vi "cRIO_4DOF_Admittance_control_v11_NewMousetrack.vi"() -> ()   [LabVIEW 2019]
uses:
  <vilib>/Platform/TimedLoop/XDataNode/timing_clust.ctl
  <vilib>/Platform/TimedLoop/XDataNode/nitl_modes.ctl
  <vilib>/Platform/TimedLoop/XDataNode/wakeup.ctl
  <vilib>/Analysis/baseanly.llb/Mean (DBL).vi
  Global 1.vi
  <vilib>/addons/control/pid/pid.llb/PID (DBL Array).vi
  <vilib>/imath/engines/lvmath2/RunTimeEngine/ArithmeticOperatorToken/NIMS_ArithmeticOperator_multmx(M,CV).vi
  <instcachedir>/0/NIMS_ArithmeticOperator_multmx(M,CV)_1D61EED49E1847F3B05DBB8EDD2FBF8F.lvgen/NIMS_ArithmeticOperator_multmx(M,CV)_1D61EED49E1847F3B05DBB8EDD2FBF8F_000.vi
  <vilib>/imathl/engines/lvmath/Functions/Error Handling/Create Error.vi
  <vilib>/imath/engines/lvmath2/RunTimeEngine/NodeEndStatement/NIMS_NodeEndStatement_Output.vi
  <instcachedir>/0/NIMS_NodeEndStatement_Output_53EC0D466D134D7ABD903AC30B43404B.lvgen/NIMS_NodeEndStatement_Output_53EC0D466D134D7ABD903AC30B43404B_002.vi
  <vilib>/imath/engines/lvmath2/RunTimeEngine/ErrorHandling/NIMS_Finalize Error.vi
  <instcachedir>/0/NIMS_NodeEndStatement_Output_53EC0D466D134D7ABD903AC30B43404B.lvgen/NIMS_NodeEndStatement_Output_53EC0D466D134D7ABD903AC30B43404B_001.vi
  <vilib>/imath/engines/lvmath2/RunTimeEngine/BuiltInFunctions/inv/NIMS_inv(GM).vi
  <instcachedir>/0/NIMS_inv(GM)_A6DF8FE880224208AACFE4CF9F659502.lvgen/NIMS_inv(GM)_A6DF8FE880224208AACFE4CF9F659502_000.vi
  <vilib>/imath/engines/lvmath2/RunTimeEngine/ErrorHandling/NIMS_Create Error From Enums.vi
  <vilib>/imath/engines/lvmath2/RunTimeEngine/IndexRead/NIMS M(R2,S).vi
  <instcachedir>/0/NIMS M(R2,S)_56813DCFDD5A484292D2195AF15D2BF5.lvgen/NIMS M(R2,S)_56813DCFDD5A484292D2195AF15D2BF5_000.vi
  <vilib>/imath/engines/lvmath2/RunTimeEngine/IndexRead/NIMS M(S,S).vi
  <instcachedir>/0/NIMS M(S,S)_AC51E74150A542F7991B9634C66F3096.lvgen/NIMS M(S,S)_AC51E74150A542F7991B9634C66F3096_000.vi
  <instcachedir>/0/NIMS_NodeEndStatement_Output_53EC0D466D134D7ABD903AC30B43404B.lvgen/NIMS_NodeEndStatement_Output_53EC0D466D134D7ABD903AC30B43404B_005.vi
  <vilib>/imath/engines/lvmath2/RunTimeEngine/BuiltInFunctions/round/NIMS_round(DBL-S).vi
  <vilib>/imath/engines/lvmath2/RunTimeEngine/BuiltInFunctions/all/NIMS_all(GS).vi
  <vilib>/imath/engines/lvmath2/RunTimeEngine/ArithmeticOperatorToken/NIMS_ArithmeticOperator_minus.vi
  <instcachedir>/0/NIMS_ArithmeticOperator_minus_12BFF9710EA5430A9EE87C5BC3F65186.lvgen/NIMS_ArithmeticOperator_minus_12BFF9710EA5430A9EE87C5BC3F65186_003.vi
  <vilib>/imath/engines/lvmath2/RunTimeEngine/ArithmeticOperatorToken/NIMS_ArithmeticOperator_power(S).vi
  <instcachedir>/0/NIMS_ArithmeticOperator_power(S)_F1497A2DE3CE4E82B2C3646D59904248.lvgen/NIMS_ArithmeticOperator_power(S)_F1497A2DE3CE4E82B2C3646D59904248_014.vi
  <vilib>/imath/engines/lvmath2/RunTimeEngine/BuiltInFunctions/cross/NIMS_cross(GV,GV).vi
  <instcachedir>/0/NIMS_cross(GV,GV)_6F1F1C643EFF41C8A983D972A94A5A15.lvgen/NIMS_cross(GV,GV)_6F1F1C643EFF41C8A983D972A94A5A15_000.vi
  <vilib>/imath/engines/lvmath2/RunTimeEngine/IndexRead/NIMS M(S).vi
  <instcachedir>/0/NIMS M(S)_B826C018497E4940AE96BD27B540B6FB.lvgen/NIMS M(S)_B826C018497E4940AE96BD27B540B6FB_000.vi
  <vilib>/imath/engines/lvmath2/RunTimeEngine/BuiltInFunctions/norm/NIMS_norm(GM,DBL).vi
  <instcachedir>/0/NIMS_norm(GM,DBL)_8BCB088F207E48DF95CF5C1DC502F84D.lvgen/NIMS_norm(GM,DBL)_8BCB088F207E48DF95CF5C1DC502F84D_000.vi
  <vilib>/imath/engines/lvmath2/RunTimeEngine/BuiltInFunctions/norm/NIMS_norm(GV,DBL).vi
  <instcachedir>/0/NIMS_norm(GV,DBL)_4A8B6F23BC0A47549B8AB805006257D9.lvgen/NIMS_norm(GV,DBL)_4A8B6F23BC0A47549B8AB805006257D9_000.vi
  <vilib>/imath/engines/lvmath2/RunTimeEngine/BuiltInFunctions/dot/NIMS_dot(GM,GM,12).vi
  <instcachedir>/0/NIMS_dot(GM,GM,12)_05F0B1C82C6743E4843530F9B3085698.lvgen/NIMS_dot(GM,GM,12)_05F0B1C82C6743E4843530F9B3085698_000.vi
  <vilib>/imath/engines/lvmath2/RunTimeEngine/IndexRead/NIMS V(S).vi
  <instcachedir>/0/NIMS V(S)_0488751826AF41519A22953C041130DC.lvgen/NIMS V(S)_0488751826AF41519A22953C041130DC_000.vi
  <vilib>/platform/TimedLoop/XDataNode/XDataNode.xnode
  <resource>/objmgr/ni.dex.rc
  <vilib>/addons/control/pid/NI_PID_pid.lvlib
  <vilib>/Analysis/NI_AALBase.lvlib
  <vilib>/Platform/TimedLoop/XDataNode/XDNodeRunTimeDep.lvlib
panel:
  in  "Sound":bool
  out "Number of laps":i16
  in  "Loop offset":dbl=0.122 format="%#_13g"
  in  "Rentry":dbl=0.08
  out "entry_cen":dbl[](array[numeric])
  out "Rexit":dbl
  out "exit_cen":dbl[](array[numeric])
  in  "Loop radius":dbl=0.127 format="%#_13g"
  in  "Manual \npulse low":bool
  in  "Global offset":dbl[](array[numeric])=[0.0, 0.0, 0.0, 0.0]
  in  "Manual \npulse high":bool
  out "SynPulseOn":bool
  in  "RunOnceLatch":bool
  out "Sync_pulse":i32
  out "Data syncing":bool
  in  "Mouse YStop":dbl=-0.33 format="%#_13g"
  out "Rmag":dbl
  out "Mousetrack ON":bool
  in  "End Wheel":bool
  in  "Begin Wheel":bool
  in  "Ftrans":bool=TRUE
  out "TransF":dbl[](array[numeric])
  in  "d_{1}_{2} (mm)":dbl[](array[numeric])=[10.0, 0.0, 0.0]
  in  "Disable X":bool
  in  "Vector correction":bool=TRUE
  in  "manual homing stop":bool
  out "c_applied":dbl[][](array[numeric])
  out "m_applied":dbl[][](array[numeric])
  out "Jostick offset":dbl[](array[numeric])
  out "Pos":dbl[](array[numeric])
  out "targetpos":dbl[](array[numeric])
  out "Rotz":dbl[][](array[numeric])
  in  "Mousetrack on":bool
  out "Loop_L":bool
  out "F":dbl[](array[numeric])
  in  "number Fsamples":i32=10
  out "Homed":bool[](array[boolean])
  out "Hall voltages":dbl[](array[numeric])
  in  "Joint offset":dbl[](array[numeric])
  in  "Target HallV":dbl[](array[numeric])=[0.1, 0.1, 0.1]
  out "Raw voltages":dbl[](array[numeric])
  in  "Record to current file":bool
  in  "Close file and open new file":bool
  in  "Stop raspberry pi":bool
  out "changes from \nadmittance {m}":dbl[](array[numeric])
  out "Joystick input":dbl[](array[numeric])
  in  "Joystick control on":bool
  out "Z position":T1(graph)
  out "Loop_R":bool
  out "Trajectory changes in Yaw":T1(graph)
  in  "Mouse force limits":dbl[](array[numeric])=[0.2, 0.2, 0.0, 0.025]
  out "loop":i32
  in  "Disable Yaw forces":bool=TRUE
  in  "Admittance scale":dbl[](array[numeric])=[1.0, 1.0, 0.0, 1.0]
  out "velocity \n(mouseframe)":dbl[](array[numeric])
  in  "RETURN TO HOME \nPOSITION AND STOP":bool
  out "Straight":bool
  in  "deltapos":dbl[](array[numeric]) format="%#_13g"
  in  "delpos limits (+/-) \ntrajectory control\n(global frame)":dbl[](array[numeric])=[0.002, 0.002, 0.0, 0.02]
  in  "delpos limits (+/-)\nadmittance control \n(mouse frame)":dbl[](array[numeric])=[0.0015, 0.0002, 0.0, 0.01]
  in  "lower limit":dbl[](array[numeric])=[-0.3, -0.34, -0.782, -6000.0]
  in  "upper limit":dbl[](array[numeric])=[0.3, 0.18, -0.65, 6000.0]
  in  "Trajectory scale":dbl[](array[numeric])=[0.05, 0.05, 0.0, 0.05]
  out "Trajectory changes in XY":T1(graph)
  in  "Disable Y forces":bool=TRUE
  out "changes from trajectory":dbl[](array[numeric])
  in  "Y_trajectory":bool
  in  "Disable -X":bool=TRUE
  out "Mousetrack_switch":bool
  in  "Yaw":dbl(slide) scale=0.0..3.142
  in  "Z":dbl(slide)=-0.7034810126582278 scale=-0.1..0.1
  in  "Y":dbl(slide)=0.05 scale=-0.3..0.05
  in  "X":dbl(slide) scale=0.0..0.06
  in  "Yaw_tajectory":bool
  out "target position":dbl[](array[numeric])
  in  "Fsense deadband\n (Nm or N)":dbl[](array[numeric])=[0.025, 0.025, 0.025, 0.001]
  in  "Output range (PWM)":cluster{"output high":dbl, "output low":dbl}[](array[cluster])=[{"output high"=100.0, "output low"=-100.0}] {"output low" format="%.2f"; "output high" format="%.2f"}
  in  "Admittance PID gains":T2(array[cluster])=[{"proportional gain (Kc)"=1.0, "integral time (Ti, min)"=0.01, "derivative time (Td, min)"=0.0}] {"derivative time (Td, min)" format="%.3f"; "integral time (Ti, min)" format="%.3f"; "proportional gain (Kc)" format="%.3f"}
  in  "Manual force":bool
  in  "Manual forces\n(mouse frame)":dbl[](array[numeric])=[0.0, 0.0, 0.0, 0.0, 0.0, 0.0]
  in  "goniometer PWM\n offset":dbl=50.0
  in  "delta PWM offset":dbl[](array[numeric])=[50.0, 50.0, 50.0]
  in  "manual position\n(global frame)":dbl[](array[numeric])=[0.0, 0.0, 0.0, 0.0, 0.0, 0.0]
  in  "Manual position control":bool
  out "Forces (N) 2":T3(graph)
  out "Torques (Nm) 2":T3(graph)
  in  "Measure Fsensor \nV offset":bool
  out "Sensor V offset":dbl[](array[numeric])
  out "Mouse forces":dbl[](array[numeric])
  in  "Out of range":bool
  out "F_measured":dbl[](array[numeric])
  out "velocity\n(global frame)":dbl[](array[numeric])
  out "Admittance changes in Yaw":T3(graph)
  out "Admittance changes in XY":T3(graph)
  out "Torques (Nm)":T3(graph)
  out "Forces (N)":T3(graph)
  in  "m":dbl[][](array[numeric])=[[0.02, 0.0, 0.0, 0.0], [0.0, 0.02, 0.0, 0.0], [0.0, 0.0, 0.30000000000000004, 0.0], [0.0, 0.0, 0.0, 2e-05]]
  in  "c":dbl[][](array[numeric])=[[0.5, 0.0, 0.0, 0.0], [0.0, 0.2, 0.0, 0.0], [0.0, 0.0, 2.0, 0.0], [0.0, 0.0, 0.0, 0.0002]]
  out "True loop time (ms)":u32
  in  "theta6":dbl
  in  "theta1,2,3 pos2":dbl=-0.75
  in  "Initial pos 2":bool
  in  "Theta PID gains":T2(array[cluster])=[{"proportional gain (Kc)"=1.0, "integral time (Ti, min)"=0.01, "derivative time (Td, min)"=0.0}] {"derivative time (Td, min)" format="%.3f"; "integral time (Ti, min)" format="%.3f"; "proportional gain (Kc)" format="%.3f"}
  in  "Theta output range":cluster{"output high":dbl, "output low":dbl}[](array[cluster])=[{"output high"=100.0, "output low"=-100.0}] {"output low" format="%.2f"; "output high" format="%.2f"}
  in  "theta 6":dbl
  in  "theta1,2,3":dbl=-0.75
  in  "Stop Joint space control":bool
  in  "Disable PID":bool
  out "velocity \n(joint space)":dbl[](array[numeric])
  out "op-space pos\n(global frame)":dbl[](array[numeric])
  out "alpha beta gamma":T1(graph)
  out "PWM":T4(graph)
  out "XY position":T1(graph)
  out "discriminant (>0)":dbl
  in  "Loop time (ms)":i64=10
  out "Data output":dbl[][](array[numeric])
  out "network stream":errorcluster
  out "Available Elements for Writing in network stream":i32
  in  "STOP saving data set":bool
  in  "PAUSE ms to wait":u32=5000
  in  "PAUSE saving data set":bool
  in  "BEGIN saving new data set":bool
  out "J":dbl[][](array[numeric])
  out "Joint_pos (rad)":dbl[](array[numeric])
  # "VALUE USED FOR INITIALISATION, TROUBLESHOOTING AND ANALYSIS"
  # "Must start USB6211DAQ.vi to read voltages from force sensor"
  # "Data saving. 'Write data to tdms file (PC VI).vi' must be started\n BEFORE this vi in order for the network stream to open correctly.\nMake sure 'Write data to tdms file (PC VI).vi' is configured correctly"
  # "Initialise system; both buttons must be pressed sequentially, left then right. Press Stop JSC when AB offset = Joint_pos"
  # "STOP AND RETURN TO HOME"
  # "VELOCITY LIMITS NB: delpos*100 = max velocity"
  # "Trajectory control. Push these buttons after manually moving the headstage to X,Y=0 m, yaw = 3.142 rad"
  # "Use Manual position control to set up or adjust the headstage position; the sliders ADD ON to the current position."
  # "POSITION LIMITS"
  # "NB: if True loop time does not equal Loop time\nthen the virtual admittance will not be correct"
  # "Admittance control. Manual position control must be switched OFF for Admittance control to work."
  # "Trajectory parameters"
  # "IR camera control: record should \nremain on while recording; close \nfile and open new for each mouse"
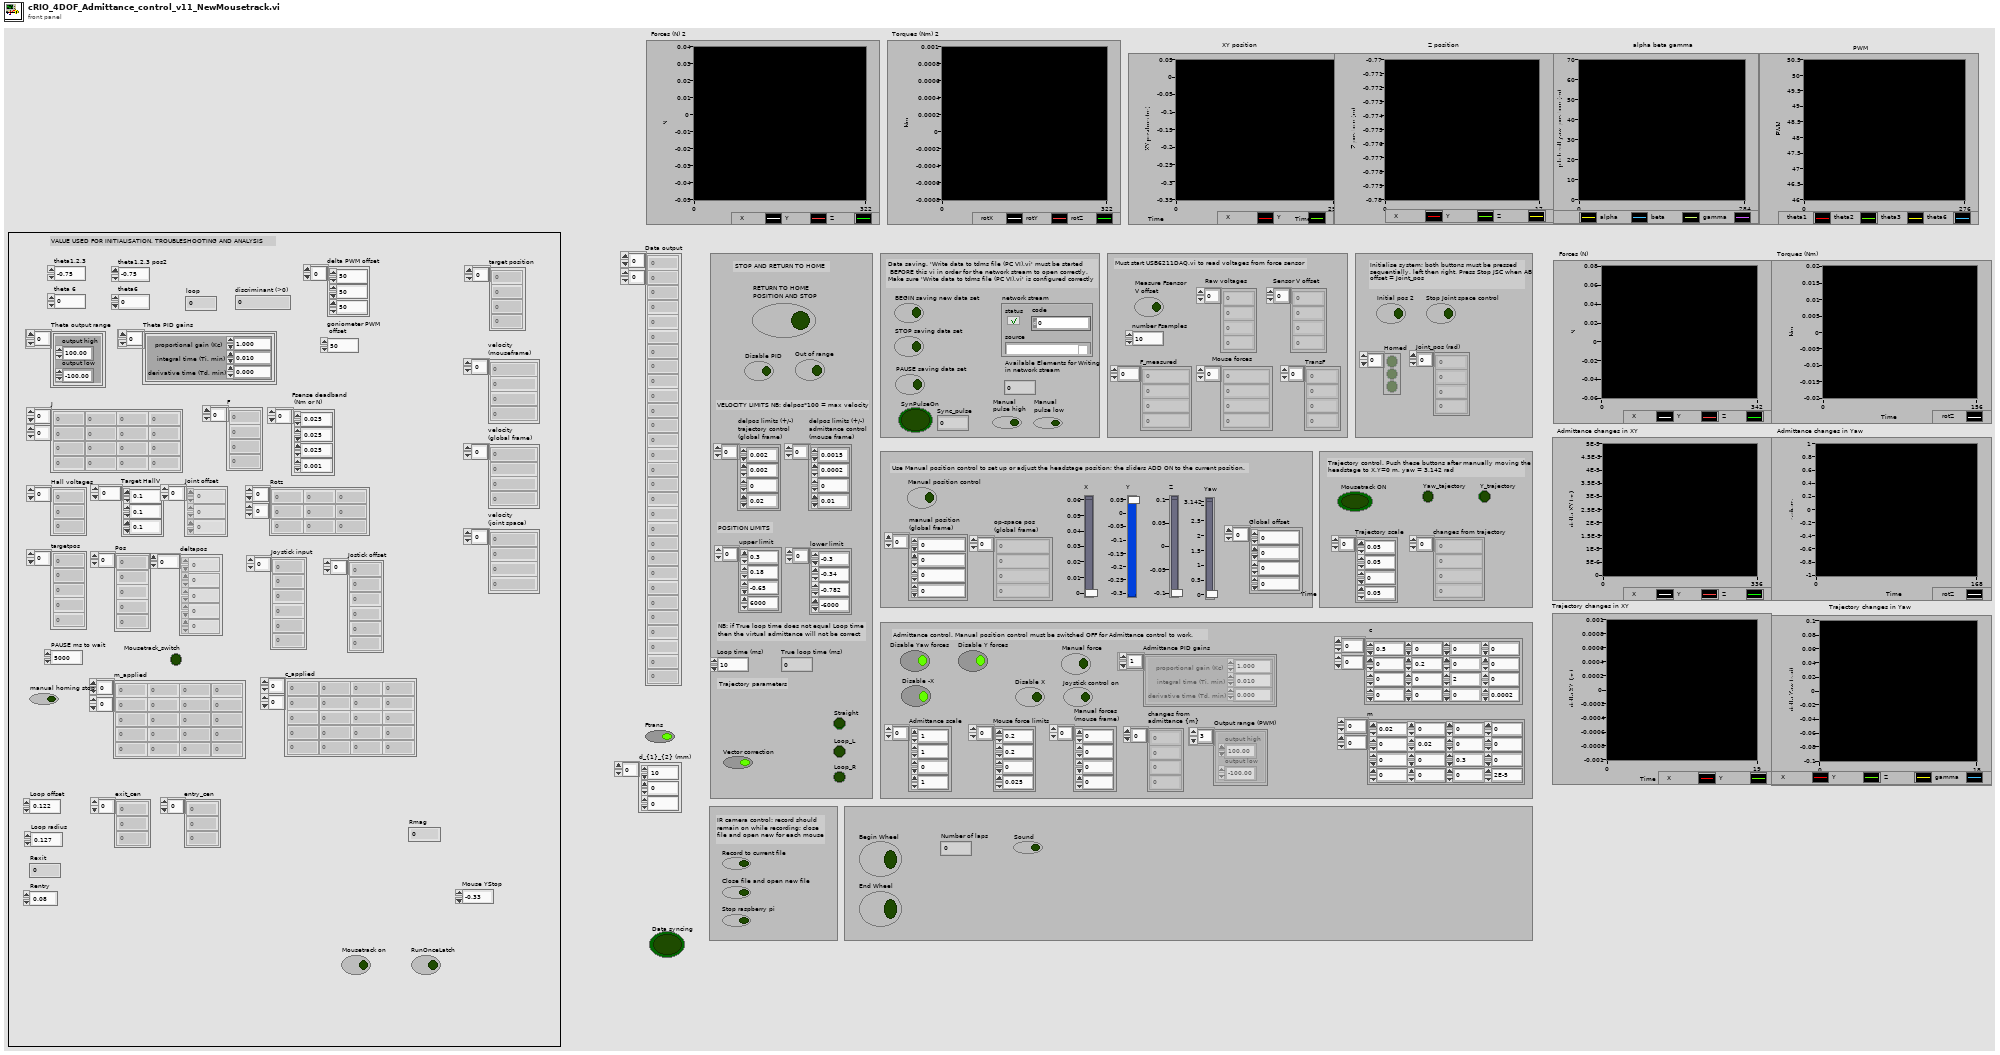
[diagram p1: front panel]
types:
  T1 = cluster{"Joint_pos (rad)[0]":dbl, "Joint_pos (rad)[1]":dbl, "Joint_pos (rad)[2]":dbl, "Joint_pos (rad)[3]":dbl, "Joint_pos (rad)[4]":dbl, "Joint_pos (rad)[5]":dbl, "Joint_pos (rad)[6]":dbl, "Joint_pos (rad)[7]":dbl, "Joint_pos (rad)[8]":dbl}
  T2 = cluster{"proportional gain (Kc)":dbl, "integral time (Ti, min)":dbl, "derivative time (Td, min)":dbl}[]
  T3 = cluster{"F[0]":dbl, "F[1]":dbl, "F[2]":dbl, "F[3]":dbl, "F[4]":dbl, "F[5]":dbl, "F[6]":dbl, "F[7]":dbl, "F[8]":dbl}
  T4 = cluster{"[0]":dbl, "[1]":dbl, "[2]":dbl, "[3]":dbl, "[4]":dbl, "[5]":dbl, "[6]":dbl, "[7]":dbl, "[8]":dbl}
  T5 = typedef "XDNodeRunTimeDep.lvlib/timing_clust.ctl" = cluster{"Expected End [f-1]":u64, "Actual End [f-1]":u64, "Finished Late? [f-1]":bool, "Expected End [i-1]":u64, "Actual End [i-1]":u64, "Finished Late? [i-1]":bool, "Expected Start [i]":u64, "Actual Start [i]":u64, "Expected Start [f]":u64, "Actual Start [f]":u64, "Source Name":string, "Structure Name":string, "Period":i64, "Deadline":i64, "Offset":i64, "Start":i64, "Priority":i32, "Timeout":i32, "Mode":T6, "Wakeup Reason":T7, "Error":errorcluster, "Source Type":string, "Secondary Source Type":string, "Global End Time":u64, "Global Start Time":u64, "Frame Duration":u64, "Iteration Duration":u64, "Assigned CPU":i32, "I/O Scan Engine Mode":u32}
  T6 = typedef "XDNodeRunTimeDep.lvlib/nitl_modes.ctl" = enum32{"No Change", "Process missed periods, maintain original phase", "Discard missed periods, maintain original phase", "Process missed periods, ignore original phase", "Discard missed periods, ignore original phase"}
  T7 = typedef "XDNodeRunTimeDep.lvlib/wakeup.ctl" = enum32{"Normal", "Aborted", "Asynchronous wakeup", "Timing source error", "Timed loop error", "Timeout"}
  T8 = cluster{"op-space pos\n(global frame)[0]":dbl, "op-space pos\n(global frame)[1]":dbl, "op-space pos\n(global frame)[2]":dbl, "op-space pos\n(global frame)[3]":dbl, "op-space pos\n(global frame)[4]":dbl, "op-space pos\n(global frame)[5]":dbl, "op-space pos\n(global frame)[6]":dbl, "op-space pos\n(global frame)[7]":dbl, "op-space pos\n(global frame)[8]":dbl}
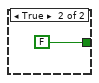
[diagram p2: hidden frame]
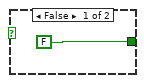
[diagram p3: hidden frame]
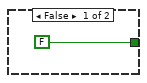
[diagram p4: hidden frame]
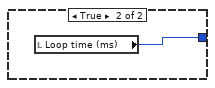
[diagram p6: hidden frame]
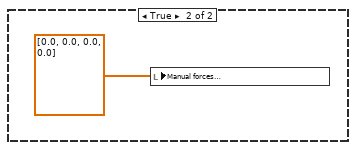
[diagram p7: hidden frame]
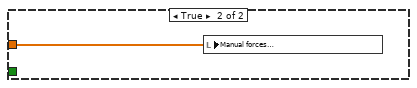
[diagram p8: hidden frame]
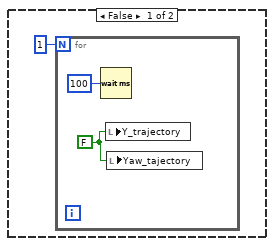
[diagram p10: hidden frame]
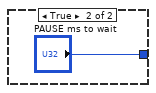
[diagram p12: hidden frame]
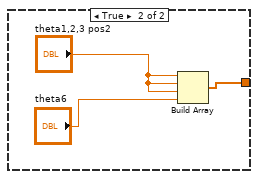
[diagram p13: hidden frame]
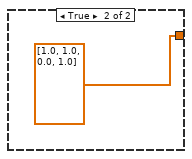
[diagram p15: hidden frame]
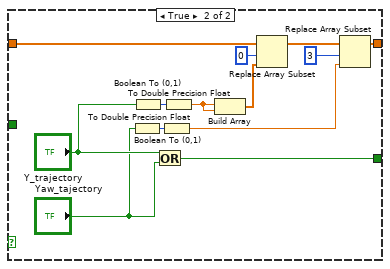
[diagram p16: hidden frame]
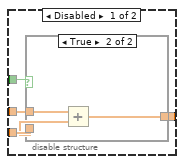
[diagram p19: hidden frame]
diagram:
  n1 = flat-sequence {
    frame #0 {
      n2 = local write "RunOnceLatch"(TRUE ("RunOnceLatch")) -> ()
    }
    frame #1 {
      n3 = while {
        stop <- FALSE stop-if-true
        n4 = flat-sequence {
          frame #0 {
            n5 = while {
              stop <- w11 stop-if-true
              n6 = local read "Mousetrack on"() -> (w10:bool)
              n7 = local read "Begin Wheel"() -> (w8:bool)
              n8 = Not(x=w10) -> (.not. x?=w9:bool)
              n9 = Wait (ms)(milliseconds to wait=u32 250) -> ()  [unwired: 1 out]
              n10 = Compound Arithmetic op=AND(w8, w9, "RunOnceLatch") -> (w11:bool)
            }
          }
          frame #1 {
            n11 = while {
              stop <- w22 stop-if-true
              n12 = local read "op-space pos\n(global frame)"() -> (w26:dbl[])
              n13 = local write "Disable Yaw forces"(TRUE ("Disable Yaw forces")) -> ()
              n14 = local write "Disable Y forces"(TRUE ("Disable Y forces")) -> ()
              n15 = mathscript code="xpos = Pos(1,1);\nypos = Pos(1,2);\nzpos = Pos(1,3);\nyawpos = Pos(1,4);\n\nxtarg = 0;\nyawtarg = pi/2;\n\ntargetpos = [xtarg, ypos, zpos, yawtarg];\n\ndelpos = real(targetpos - Pos);"("Pos"=w26) -> ("delpos"=w21:dbl[])  [unwired: 1 in, 1 out]
              n16 = local write "Disable -X"(TRUE ("Disable -X")) -> ()
              n17 = local write "delpos limits (+/-)\nadmittance control \n(mouse frame)"(dbl[] [0.0008, 0.0002, 0.0, 0.01] ("delpos limits (+/-)\nadmittance control \nDzone")) -> ()
              n18 = local read "op-space pos\n(global frame)"() -> (w24:dbl[])
              n19 = local read "entry_cen"() -> (w14:dbl[])
              n20 = Index Array(array=w24, index=1) -> (element=w23:dbl)
              n21 = Index Array(array=w14, index=1) -> (element=w13:dbl)
              n22 = Greater?(x=w23, y=w13) -> (0:w22:bool)
              n23 = local write "deltapos"(w21) -> ()
              n24 = Wait (ms)(milliseconds to wait=u32 10) -> ()  [unwired: 1 out]
            }
          }
          frame #2 {
            n25 = while {
              stop <- w167 stop-if-true
              n26 = local read "entry_cen"() -> (w174:dbl[])
              n27 = local read "Rentry"() -> (w173:dbl)
              n28 = local read "op-space pos\n(global frame)"() -> (w166:dbl[])
              n29 = local read "entry_cen"() -> (w165:dbl[])
              n30 = local read "op-space pos\n(global frame)"() -> (w172:dbl[])
              n31 = mathscript code="xpos = Pos(1,1);\nypos = Pos(1,2);\nzpos = Pos(1,3);\nyawpos = Pos(1,4);\n\nRotz = [cos(yawpos),-sin(yawpos),0; sin(yawpos),cos(yawpos),0; 0,0,1];\nxhat = [1, 0, 0]';\nzhat = [0, 0, 1]';\n\nRLsgn = 1;   % clockwise\n\nxcen = xpos - w_cen(1);\nycen = ypos - w_cen(2);\nRmag = real((xcen^2 + ycen^2)^0.5);\nxtarg = R/Rmag*xcen  + w_cen(1);\nytarg = R/Rmag*ycen + w_cen(2);      \n\nvecpos = [xcen, ycen, 0]';         % position vector, zero'd circle\nvecyaw = RLsgn*cross(vecpos,zhat);  % yaw vector\nvecyaw_o = Rotz'*vecyaw;        %  yaw vector transformed by actual yaw\nyawerrsign = sign(0 - vecyaw_o(2));  % sign of yaw error\nyawerrmag = acos(dot(vecyaw_o,xhat)/(norm(vecyaw_o)*norm(xhat))); % magnitude of yaw error   \nyawtarg  = yawpos - yawerrsign*real(yawerrmag); % target yaw position\n\ntargetpos = [xtarg, ytarg, zpos, yawtarg];\n\ndelpos = real(targetpos - Pos);"("Pos"=w172, "R"=w173, "w_cen"=w174) -> ("delpos"=w164:dbl[])  [unwired: 1 in, 2 out]
              n32 = Index Array(array=w166, index=0) -> (element=w170:dbl)
              n33 = Index Array(array=w165, index=0) -> (element=w168:dbl)
              n34 = Greater?(x=w170, y=w168) -> (0:w167:bool)
              n35 = local write "deltapos"(w164) -> ()
            }
          }
          frame #3 {
            n36 = Wait (ms)(milliseconds to wait=u32 10) -> ()  [unwired: 1 out]
            n37 = local write "RunOnceLatch"(FALSE ("RunOnceLatch")) -> ()
            n38 = local write "Mousetrack on"(TRUE ("Eight maze on")) -> ()
            n39 = local write "Begin Wheel"(FALSE ("Begin Wheel")) -> ()
          }
        }
      }
    }
  }
  n40 = flat-sequence {
    frame #0 {
      w610 = 0.0 ("X")
      n41 = local write "RETURN TO HOME \nPOSITION AND STOP"(FALSE ("RETURN TO HOME \nPOSITION AND STOP")) -> ()
      n42 = local write "Joystick control on"(FALSE ("Joystick control on")) -> ()
      n43 = local write "Initial pos 2"(FALSE ("Initial pos 2")) -> ()
      n44 = local write "Stop Joint space control"(FALSE ("Stop Joint space control")) -> ()
      n45 = local write "Disable PID"(TRUE ("Disable PID")) -> ()
      n46 = local write "Manual force"(FALSE ("Manual force")) -> ()
      n47 = local write "Manual \npulse high"(FALSE ("Manual pulse high")) -> ()
      n48 = local write "Manual position control"(TRUE ("Manual velocity control")) -> ()
      n49 = local write "Begin Wheel"(FALSE ("Begin Wheel")) -> ()
      n50 = local write "Disable PID"(FALSE ("Enable PID")) -> ()
      n51 = local write "Mousetrack on"(FALSE ("Trajectory control")) -> ()
      n52 = local write "Yaw_tajectory"(FALSE ("Mousetrack_Yaw")) -> ()
      n53 = local write "Y_trajectory"(FALSE ("Mousetrack_Yaw")) -> ()
      n54 = local write "Manual \npulse low"(FALSE ("Manual pulse high")) -> ()
      n55 = shared-variable "RT CompactRIO Target\\Mod7\\DIO0"(FALSE ("DIO0")) -> ()  [unwired: 1 in, 1 out]
      n56 = local write "theta1,2,3 pos2"(-0.25 ("theta1,2,3 pos2")) -> ()
      n57 = local write "theta1,2,3"(-0.75 ("theta1,2,3")) -> ()
      n58 = global write "Global 1.vi" "a_1 (m)"(0.1 ("a_4 (m)")) -> ()
      n59 = local write "Manual forces\n(mouse frame)"(dbl[] [0.0, 0.0, 0.0, 0.0] ("Manual forces")) -> ()
      n60 = local write "Yaw"(w610) -> ()
      n61 = local write "theta6"(0.0 ("theta4,5,6")) -> ()
      n62 = global write "Global 1.vi" "Rf (m)"(0.1898 ("Rf (m)")) -> ()
      n63 = global write "Global 1.vi" "Ld (m)"(0.656 ("Ld (m)")) -> ()
      n64 = global write "Global 1.vi" "L6 (m)"(0.22 ("a_4 (m)")) -> ()
      n65 = global write "Global 1.vi" "Rm (m)"(0.1 ("Rm (m)")) -> ()
      n66 = global write "Global 1.vi" "Lp (m)"(0.34 ("Lp (m)")) -> ()
      n67 = local write "Global offset"(dbl[] [-0.003, 0.0, 0.0, 0.0] ("Global offset")) -> ()
      n68 = local write "Y"(w610) -> ()
      n69 = local write "X"(w610) -> ()
      n70 = local write "Z"(w610) -> ()
      n71 = local write "Close file and open new file"(FALSE ("Close file and open new file")) -> ()
      n72 = local write "Record to current file"(FALSE ("Record to current file")) -> ()
      n73 = local write "Stop raspberry pi"(FALSE ("Stop raspberry pi")) -> ()
      n74 = local write "Target HallV"(dbl[] [0.1, 0.1, 0.1] ("Joint offset")) -> ()
      n75 = local write "Theta output range"(cluster{"output high":dbl, "output low":dbl}[] [{"output high"=50.0, "output low"=-50.0}] ("XYZ output range")) -> ()
      n76 = local write "Theta PID gains"(T2 [{"proportional gain (Kc)"=10.0, "integral time (Ti, min)"=0.0, "derivative time (Td, min)"=0.0}] ("XYZ PID gains")) -> ()
      n77 = local write "Admittance PID gains"(T2 [{"proportional gain (Kc)"=80.0, "integral time (Ti, min)"=0.5, "derivative time (Td, min)"=0.0}, {"proportional gain (Kc)"=80.0, "integral time (Ti, min)"=0.5, "derivative time (Td, min)"=0.0}, {"proportional gain (Kc)"=40.0, "integral time (Ti, min)"=0.5, "derivative time (Td, min)"=0.0}, {"proportional gain (Kc)"=200.0, "integral time (Ti, min)"=0.0, "derivative time (Td, min)"=0.0}] ("XYZ PID gains")) -> ()
      n78 = local write "Output range (PWM)"(cluster{"output high":dbl, "output low":dbl}[] [{"output high"=50.0, "output low"=-50.0}, {"output high"=50.0, "output low"=-50.0}, {"output high"=50.0, "output low"=-50.0}, {"output high"=50.0, "output low"=-50.0}] ("XYZ output range")) -> ()
      n79 = local write "upper limit"(dbl[] [0.3, 0.18, -0.65, 6000.0] ("upper limit")) -> ()
      n80 = local write "lower limit"(dbl[] [-0.3, -0.34, -0.782, -6000.0] ("lower limit")) -> ()
    }
    frame #1 {
      n81 = while {
        stop <- w634 stop-if-true
        w644 = dbl[] [50.0, 50.0, 50.0]  # PWM 50% offset
        n82 = shared-variable "RT CompactRIO Target\\Mod8\\AI28"() -> (w652:dbl)  [unwired: 1 in, 1 out]
        n83 = shared-variable "RT CompactRIO Target\\Mod8\\AI27"() -> (w651:dbl)  [unwired: 1 in, 1 out]
        n84 = shared-variable "RT CompactRIO Target\\Mod8\\AI20"() -> (w653:dbl)  [unwired: 1 in, 1 out]
        n85 = Build Array(w653, w652, w651) -> (w640:dbl[])
        "Hall voltages" <- w640
        n86 = call-poly <vilib>:"PID.vi"("output range"=cluster{"output high":dbl, "output low":dbl}[] [{"output high"=5.0, "output low"=-5.0}], "PID gains"=T2 [{"proportional gain (Kc)"=4.0, "integral time (Ti, min)"=0.0, "derivative time (Td, min)"=0.0}], "process variable"=w640, "setpoint"="Target HallV") -> ("output"=w637:dbl[])  [unwired: 6 in, 1 out]
        n87 = Negate(x=w637) -> (-x=w636:dbl[])
        n88 = Add(x=w636, y=w644) -> (x+y=w643:dbl[])
        n89 = Add(x=dbl[] [0.05, 0.05, 0.05], y="Target HallV") -> (x+y=w639:dbl[])
        n90 = Subtract(x="Target HallV", y=dbl[] [0.0, 0.0, 0.0]) -> (x-y=w630:dbl[])
        n91 = Index Array(array=w643, index=1) -> (element=w646:dbl)
        n92 = Index Array(array=w643, index=0) -> (element=w647:dbl)
        n93 = Index Array(array=w643, index=2) -> (element=w645:dbl)
        n94 = In Range and Coerce(upper limit=w639, x=w640, lower limit=w630) -> (In Range?=w638:bool[])  [unwired: 1 out]
        "Homed" <- w638
        n95 = And Array Elements(Boolean array=w638) -> (logical AND=w635:bool)
        n96 = In Range and Coerce(upper limit=52.0, x=w647, lower limit=48.0) -> (coerced(x)=w656:dbl)  [unwired: 1 out]
        n97 = In Range and Coerce(upper limit=52.0, x=w646, lower limit=48.0) -> (coerced(x)=w655:dbl)  [unwired: 1 out]
        n98 = In Range and Coerce(upper limit=52.0, x=w645, lower limit=48.0) -> (coerced(x)=w654:dbl)  [unwired: 1 out]
        n99 = Or(x=w635, y="manual homing stop") -> (x .or. y?=w634:bool)
        n100 = shared-variable "RT CompactRIO Target\\Mod5\\PWM1"(w655) -> ()  [unwired: 1 in, 1 out]
        n101 = shared-variable "RT CompactRIO Target\\Mod5\\PWM2"(w654) -> ()  [unwired: 1 in, 1 out]
        n102 = shared-variable "RT CompactRIO Target\\Mod5\\PWM0"(w656) -> ()  [unwired: 1 in, 1 out]
      }
    }
    frame #2 {
      n103 = call "cRIO_4DoF_Encoders_counts2rad(subVI).vi"() -> ("Theta3"=w664:dbl, "Theta2"=w665:dbl, "Theta1"=w666:dbl, "Theta6"=w667:dbl)  [unwired: 4 in]
      n104 = Build Array(w666, w665, w664, w667) -> (w663:dbl[])
      n105 = local write "Joint offset"(w663) -> ()
    }
    frame #3 {
      n106 = while "Joint space control" {
        stop <- w675 stop-if-true
        w678 = dbl[] [50.0, 50.0, 50.0, 50.0]  # PWM 50% offset
        n107 = case shown="False" "Initial pos 2" {
          tunnel: [w700 w701] -> w695
          frame False {
            n108 = Build Array("theta1,2,3", "theta1,2,3", "theta1,2,3", "theta 6") -> (w700:dbl[])
          }
          frame True {
            n109 = Build Array("theta1,2,3 pos2", "theta1,2,3 pos2", "theta1,2,3 pos2", "theta6") -> (w701:dbl[])
          }
        }
        n110 = local read "Joint_pos (rad)"() -> (w669:dbl[])
        n111 = call-poly <vilib>:"PID.vi"("output range"="Theta output range", "PID gains"="Theta PID gains", "process variable"=w669, "setpoint"=w695) -> ("output"=w668:dbl[])  [unwired: 6 in, 1 out]
        n112 = Add(x=w668, y=w678) -> (x+y=w677:dbl[])
        n113 = Index Array(array=w677, index=0) -> (element=w690:dbl)
        n114 = Index Array(array=w677, index=1) -> (element=w681:dbl)
        n115 = Index Array(array=w677, index=2) -> (element=w680:dbl)
        n116 = Index Array(array=w677, index=3) -> (element=w679:dbl)
        n117 = In Range and Coerce(upper limit=99.0, x=w690, lower limit=1.0) -> (coerced(x)=w673:dbl)  [unwired: 1 out]
        n118 = In Range and Coerce(upper limit=99.0, x=w681, lower limit=1.0) -> (coerced(x)=w672:dbl)  [unwired: 1 out]
        n119 = In Range and Coerce(upper limit=99.0, x=w679, lower limit=1.0) -> (coerced(x)=w670:dbl)  [unwired: 1 out]
        n120 = In Range and Coerce(upper limit=99.0, x=w680, lower limit=1.0) -> (coerced(x)=w671:dbl)  [unwired: 1 out]
        n121 = shared-variable "RT CompactRIO Target\\Mod5\\PWM2"(w671) -> ()  [unwired: 1 in, 1 out]
        n122 = shared-variable "RT CompactRIO Target\\Mod5\\PWM3"(w670) -> ()  [unwired: 1 in, 1 out]
        n123 = shared-variable "RT CompactRIO Target\\Mod5\\PWM0"(w673) -> ()  [unwired: 1 in, 1 out]
        n124 = shared-variable "RT CompactRIO Target\\Mod5\\PWM1"(w672) -> ()  [unwired: 1 in, 1 out]
        n125 = And(x="Stop Joint space control", y="Initial pos 2") -> (x .and. y?=w675:bool)
      }
    }
    frame #4 {
      w720 = dbl[] [50.0, 50.0, 50.0, 50.0] ("y")
      w726 = 0.0 ("X")
      n126 = Wait (ms)(milliseconds to wait=u32 50) -> ()  [unwired: 1 out]
      n127 = Index Array(array=w720, index=0) -> (element=w707:dbl)
      n128 = Index Array(array=w720, index=1) -> (element=w706:dbl)
      n129 = Index Array(array=w720, index=2) -> (element=w705:dbl)
      n130 = Index Array(array=w720, index=3) -> (element=w704:dbl)
      n131 = local write "Yaw"(w726) -> ()
      n132 = local write "Z"(w726) -> ()
      n133 = local write "Y"(w726) -> ()
      n134 = local write "X"(w726) -> ()
      n135 = In Range and Coerce(upper limit=99.0, x=w707, lower limit=1.0) -> (coerced(x)=w711:dbl)  [unwired: 1 out]
      n136 = In Range and Coerce(upper limit=99.0, x=w706, lower limit=1.0) -> (coerced(x)=w710:dbl)  [unwired: 1 out]
      n137 = In Range and Coerce(upper limit=99.0, x=w705, lower limit=1.0) -> (coerced(x)=w709:dbl)  [unwired: 1 out]
      n138 = In Range and Coerce(upper limit=99.0, x=w704, lower limit=1.0) -> (coerced(x)=w708:dbl)  [unwired: 1 out]
      n139 = shared-variable "RT CompactRIO Target\\Mod5\\PWM0"(w711) -> ()  [unwired: 1 in, 1 out]
      n140 = shared-variable "RT CompactRIO Target\\Mod5\\PWM1"(w710) -> ()  [unwired: 1 in, 1 out]
      n141 = shared-variable "RT CompactRIO Target\\Mod5\\PWM2"(w709) -> ()  [unwired: 1 in, 1 out]
      n142 = shared-variable "RT CompactRIO Target\\Mod5\\PWM3"(w708) -> ()  [unwired: 1 in, 1 out]
    }
    frame #5 {
      n143 = local read "op-space pos\n(global frame)"() -> (w730:dbl[])
      n144 = node-c288("Loop time (ms)") -> (w729:T5)  [unwired: 3 in]
      n145 = timed-loop {
        shift-right: [w924] -> _
        shift-left: _ -> [w923]
        shift-right: ["Manual position control"] -> _
        shift-left: FALSE ("Manual position control") -> [w891]
        shift-right: [w838] -> _
        shift-left: w730 -> [w735]
        shift-right: ["Mousetrack on"] -> _
        shift-left: _ -> [w907]
        timing: w729 -> [_]
        timing-out: [_] -> w728
        i -> [w882]
        stop <- "RETURN TO HOME \nPOSITION AND STOP" stop-if-true
        w751 = dbl[] [0.005, 0.005, 0.0, 0.1] ("upper limit")
        w807 = 3 ("index (row)")
        w808 = 1 ("index (row)")
        w809 = 3 ("index (row)")
        w810 = 1 ("index (row)")
        w880 = 0 ("index (row)")
        w881 = 0 ("index (row)")
        n146 = node-c288() -> ()  [unwired: 1 in, 1 out]
        n147 = Build Array("X", "Y", "Z", "Yaw") -> (w844:dbl[])
        n148 = local read "Joint_pos (rad)"() -> (w852:dbl[])
        n149 = Add(x="manual position\n(global frame)", y=w844) -> (x+y=w734:dbl[])
        n150 = global read "Global 1.vi" "F_measured"() -> (w775:dbl[])
        n151 = Or(x="Begin Wheel", y="End Wheel") -> (x .or. y?=w732:bool)
        n152 = case shown="False" "Mousetrack on" {
          tunnel: [w989 w997] -> w889
          tunnel: [w988 w996] -> w877
          tunnel: dbl[] [0.0, 0.0, 0.0, 0.0] ("array") -> [w990 w993]
          tunnel: w732 -> [w988 _]
          frame False {
            n153 = case shown="False" w988 {
              tunnel: w990 -> [w991 _]
              tunnel: [w991 dbl[] [1.0, 1.0, 0.0, 1.0] ("array")] -> w989
              frame False {
              }
              frame True {
              }
            }
          }
          frame True {
            n154 = Boolean To (0,1)(Boolean="Yaw_tajectory") -> (0, 1=w1004:i16)
            n155 = Boolean To (0,1)(Boolean="Y_trajectory") -> (0, 1=w1005:i16)
            n156 = Or(x="Y_trajectory", y="Yaw_tajectory") -> (x .or. y?=w996:bool)
            n157 = To Double Precision Float(number=w1004) -> (double precision float=w998:dbl)
            n158 = To Double Precision Float(number=w1005) -> (double precision float=w1002:dbl)
            n159 = Build Array(w1002, w1002) -> (w1001:dbl[])
            n160 = Replace Array Subset(array=w993, new element=w1001, index=0) -> (w999:dbl[])
            n161 = Replace Array Subset(array=w999, new element=w998, index=3) -> (w997:dbl[])
          }
        }
        n162 = Index Array(array=w735, index=1) -> (element=w740:dbl)
        n163 = mathscript code="m = -0.004/0.290;\n\nzadjust = ypos*m;"("ypos"=w740) -> ("zadjust"=w738:dbl)  [unwired: 1 in, 1 out]
        n164 = Index Array(array=w852, index=0) -> (element=w854:dbl)
        n165 = Index Array(array=w852, index=1) -> (element=w853:dbl)
        n166 = Index Array(array=w852, index=2) -> (element=w851:dbl)
        n167 = Index Array(array=w852, index=3) -> (element=w850:dbl)
        n168 = call "cRIO_4DoF_Force_conversion.vi"("Manual force"="Manual force", "F_measured"=w775, "Manual forces in"="Manual forces\n(mouse frame)") -> ("Force control"=w768:dbl[], "F_mouse"=→"Mouse forces":dbl[])  [unwired: 7 in]
        n169 = call "cRIO_4DoF_Delta_forward_kinematics.vi"("theta3"=w851, "theta2"=w853, "theta1"=w854) -> ("YD"=w857:cdb, "ZD"=w858:cdb, "discriminant (>0)"=→"discriminant (>0)":dbl, "XD"=w856:cdb)  [unwired: 5 in]
        n170 = In Range and Coerce(upper limit=0.004, x=w738, lower limit=0.0) -> (coerced(x)=w739:dbl)  [unwired: 1 out]
        n171 = case shown="True" w732 {
          tunnel: w734 -> [w957 w963]
          tunnel: w739 -> [_ w960]
          tunnel: [w957 w958] -> w733
          frame False {
          }
          frame True {
            n172 = Replace Array Subset(array=dbl[] [0.0, 0.0, 0.0, 0.0] ("y"), new element=w960, index=2) -> (w959:dbl[])
            n173 = Add(x=w963, y=w959) -> (x+y=w958:dbl[])
          }
        }
        n174 = call "cRIO_4DoF_Gonio_forward_kinematics.vi"("X in"=w856, "Y in"=w857, "Z in"=w858, "Theta6_meas"=w850) -> ("X out"=w867:dbl, "Y out"=w866:dbl, "Z out"=w865:dbl, "yaw"=w864:dbl)  [unwired: 7 in, 1 out]
        n175 = call "cRIO_4DOF_Jacobian_v3.vi"("XD"=w856, "YD"=w857, "ZD"=w858, "Joint positions"=w852) -> ("J"=w868:dbl[][])  [unwired: 7 in]
        "J" <- w868
        n176 = Multiply(x="deltapos", y=w889) -> (x*y=w887:dbl[])
        n177 = Multiply(x=w887, y="Trajectory scale") -> (x*y=w876:dbl[])
        n178 = call "cRIO_4DoF_PluckerTrans.vi"("Force control"=w768, "d_{1}_{2} (mm)"="d_{1}_{2} (mm)") -> ("TransF"=w770:dbl[])  [unwired: 9 in]
        "TransF" <- w770
        n179 = Array To Cluster(array=w876) -> (cluster=→"Trajectory changes in XY":T4)
        n180 = Build Array(w867, w866, w865, w864) -> (w749:dbl[])
        n181 = Array To Cluster(array=w876) -> (cluster=→"Trajectory changes in Yaw":T4)
        n182 = Negate(x="delpos limits (+/-) \ntrajectory control\n(global frame)") -> (-x=w896:dbl[])
        n183 = Negate(x=w751) -> (-x=w750:dbl[])
        n184 = call "cRIO_4DoF_Encoders_countsvel2radvel(subVI).vi"() -> ("Joint_space_velocity"=w830:dbl[])  [unwired: 11 in]
        "velocity \n(joint space)" <- w830
        n185 = In Range and Coerce(upper limit=w751, x="Global offset", lower limit=w750) -> (coerced(x)=w748:dbl[])  [unwired: 1 out]
        n186 = In Range and Coerce(upper limit="delpos limits (+/-) \ntrajectory control\n(global frame)", x=w876, lower limit=w896) -> (coerced(x)=w878:dbl[])  [unwired: 1 out]
        n187 = mathscript code="Joint_vel = Joint_vel';\n\nOp_vel = J*Joint_vel;\n\nOp_vel = real(Op_vel);"("J"=w868, "Joint_vel"=w830) -> ("Op_vel"=w886:dbl[][])  [unwired: 1 in, 1 out]
        n188 = case shown="True" "Ftrans" {
          tunnel: w770 -> [_ w1007]
          tunnel: [w1006 w1007] -> w769
          tunnel: w768 -> [w1006 _]
          frame False {
          }
          frame True {
          }
        }
        n189 = case shown="True" w877 {
          tunnel: [dbl[] [0.0, 0.0, 0.0, 0.0] w1027] -> w879
          tunnel: w878 -> [_ w1027]
          frame False {
          }
          frame True {
          }
        }
        "changes from trajectory" <- w879
        n190 = Greater?(x="Mousetrack on", y=w907) -> (0:w905:bool)
        n191 = Less?(x="Mousetrack on", y=w907) -> (x < y?=w906:bool)
        n192 = Less?(x=w882, y=10) -> (x < y?=w755:bool)
        n193 = Or(x=w905, y=w906) -> (x .or. y?=→"Mousetrack_switch":bool)
        n194 = Add(x=w749, y=w748) -> (x+y=w747:dbl[])
        "op-space pos\n(global frame)" <- w747
        n195 = Or(x="Manual position control", y=w755) -> (x .or. y?=w757:bool)
        n196 = call "cRIO_4DoF_Fsense_deadband(subVI).vi"("Fsense deadband (Nm or N)"="Fsense deadband\n (Nm or N)", "Enable Fsense Deadband"=TRUE, "F_{2} in"=w769) -> ("F_{2} out"=w861:dbl[])  [unwired: 8 in]
        n197 = Reshape Array(w886, 4 ("dimension size")) -> (w863:dbl[])
        "velocity\n(global frame)" <- w863
        n198 = call "cRIO_4DoF_InvYaw_global2mouse_v2.vi"("op-space pos"=w747, "op_vel"=w863) -> ("vel_out"=w834:dbl[])  [unwired: 9 in]
        "velocity \n(mouseframe)" <- w834
        n199 = Negate(x="Mouse force limits") -> (-x=w900:dbl[])
        n200 = local read "Loop time (ms)"() -> (w835:i64)
        n201 = In Range and Coerce(upper limit="Mouse force limits", x=w861, lower limit=w900) -> (coerced(x)=w836:dbl[])  [unwired: 1 out]
        n202 = call "cRIO_4DoF_Admittance_controller_v3.vi"("F"=w836, "v_2 in"=w834, "c"="c", "m"="m", "Loop time (ms)"=w835) -> ("del_m"=w837:dbl[])  [unwired: 9 in, 1 out]
        n203 = local read "op-space pos\n(global frame)"() -> (w873:dbl[])
        n204 = local read "Yaw_tajectory"() -> (w872:bool)
        n205 = local read "deltapos"() -> (w874:dbl[])
        n206 = call "cRIO_4DoF_deactivate_mouseforce_axes.vi"("Disable Yaw forces"="Disable Yaw forces", "Disable X"="Disable X", "Disable Y forces"="Disable Y forces", "Disable -X"="Disable -X", "del_m in"=w837) -> ("del_m out"=w871:dbl[])  [unwired: 6 in]
        n207 = disable-structure shown="Enabled" {
          disable-tunnel: w874 -> [w1018 _]
          disable-tunnel: w873 -> [w1017 w1023]
          disable-tunnel: w872 -> [w1016 _]
          disable-tunnel: [w1015 w1023] -> w833
          frame Disabled {
            n208 = case shown="True" w1016 {
              tunnel: w1018 -> [_ w1022]
              tunnel: w1017 -> [w1019 w1021]
              tunnel: [w1019 w1020] -> w1015
              frame False {
              }
              frame True {
                n209 = Add(x=w1022, y=w1021) -> (x+y=w1020:dbl[])
              }
            }
          }
          frame Enabled {
          }
        }
        n210 = local read "op-space pos\n(global frame)"() -> (w915:dbl[])
        n211 = Multiply(x=w871, y="Admittance scale") -> (x*y=w869:dbl[])
        n212 = Index Array(array=w833, index=3) -> (element=w831:dbl)
        n213 = Negate(x="delpos limits (+/-)\nadmittance control \n(mouse frame)") -> (-x=w898:dbl[])
        n214 = In Range and Coerce(upper limit="delpos limits (+/-)\nadmittance control \n(mouse frame)", x=w869, lower limit=w898) -> (coerced(x)=w812:dbl[])  [unwired: 1 out]
        "changes from \nadmittance {m}" <- w812
        n215 = local read "J"() -> (w912:dbl[][])
        n216 = call "cRIO_4DoF_Yaw_mouse2global_v2.vi"("yawangle"=w831, "Mouse forces"=w812) -> ("F_2"=w792:dbl[])  [unwired: 9 in]
        n217 = local read "Begin Wheel"() -> (w763:bool)
        n218 = local read "End Wheel"() -> (w761:bool)
        n219 = local read "Loop_L"() -> (w784:bool)
        n220 = local read "Loop_R"() -> (w783:bool)
        n221 = local read "op-space pos\n(global frame)"() -> (w785:dbl[])
        n222 = local read "Loop offset"() -> (w786:dbl)
        n223 = local read "Straight"() -> (w790:bool)
        n224 = Not(x=w790) -> (.not. x?=w789:bool)
        n225 = Not(x=w763) -> (.not. x?=w764:bool)
        n226 = Not(x=w761) -> (.not. x?=w760:bool)
        n227 = Compound Arithmetic op=AND("Vector correction", w789, w764, w760) -> (w787:bool)
        n228 = case shown="True" w787 {
          tunnel: w792 -> [w1008 w1011]
          tunnel: [w1008 w1009] -> w791
          tunnel: w786 -> [_ w1010]
          tunnel: w785 -> [_ w1012]
          tunnel: w784 -> [_ w1014]
          tunnel: w783 -> [_ w1013]
          frame False {
          }
          frame True {
            n229 = call "cRIO_4DoF_vectorcompensation_eightplus.vi"("F_2"=w1011, "Radius"=w1010, "op-space pos\n(global frame)"=w1012, "Loop_R"=w1013, "Loop_L"=w1014) -> ("delPosout"=w1009:dbl[])  [unwired: 6 in]
          }
        }
        n230 = Compound Arithmetic op=ADD(w735, w791, w879) -> (w911:dbl[])
        n231 = case shown="False" w757 {
          tunnel: w911 -> [w1096 _]
          tunnel: [w1095 w1107] -> w839
          tunnel: w733 -> [w1097 w1108]
          tunnel: w755 -> [_ w1103]
          tunnel: w891 -> [_ w1102]
          tunnel: "Manual position control" -> [_ w1101]
          frame False {
            w1099 = 2 ("index")
            n232 = Array Subset(array=w1097, index=w1099, length=1) -> (w1100:dbl[])
            n233 = Replace Array Subset(array=w1096, new element=w1100, index=w1099) -> (w1095:dbl[])
          }
          frame True {
            n234 = local read "Mousetrack_switch"() -> (w1104:bool)
            n235 = Greater?(x=w1101, y=w1102) -> (0:w1105:bool)
            n236 = Compound Arithmetic op=OR(w1103, w1105, w1104) -> (w1106:bool)
            n237 = case shown="False" w1106 {
              tunnel: [w1109 w1111] -> w1107
              tunnel: w1108 -> [w1109 _]
              frame False {
              }
              frame True {
                w1110 = 0.0 ("Z")
                n238 = local read "op-space pos\n(global frame)"() -> (w1111:dbl[])
                n239 = local write "manual position\n(global frame)"(w1111) -> ()
                n240 = local write "target position"(w1111) -> ()
                n241 = local write "Yaw"(w1110) -> ()
                n242 = local write "X"(w1110) -> ()
                n243 = local write "Y"(w1110) -> ()
                n244 = local write "Z"(w1110) -> ()
              }
            }
          }
        }
        n245 = In Range and Coerce(upper limit="upper limit", x=w839, lower limit="lower limit") -> (coerced(x)=w838:dbl[])  [unwired: 1 out]
        "target position" <- w838
        n246 = call-poly <vilib>:"PID.vi"("output range"="Output range (PWM)", "PID gains"="Admittance PID gains", "process variable"=w915, "setpoint"=w838) -> ("output"=w813:dbl[])  [unwired: 6 in, 1 out]
        n247 = mathscript code="opspace = [op_vel]';\njointspace = inv(J)*opspace;\nlinrad = real(jointspace(1:3,1));\nrotrad = real(jointspace(4,1));" "Velocity conversion (in PWM space)"("op_vel"=w813, "J"=w912) -> ("linrad"=w926:dbl[], "rotrad"=w929:dbl)  [unwired: 1 in, 1 out]
        n248 = Compound Arithmetic op=OR(w755, "Disable PID", "Out of range") -> (w920:bool)
        n249 = local read "c_applied"() -> (w805:dbl[][])
        n250 = local read "m_applied"() -> (w806:dbl[][])
        n251 = Add(x=w926, y="delta PWM offset") -> (x+y=w928:dbl[])
        n252 = Tick Count (ms)() -> (millisecond timer value=w754:u32)
        n253 = Add(x=w929, y="goniometer PWM\n offset") -> (x+y=w927:dbl)
        n254 = case shown="False" w920 {
          tunnel: w928 -> [w1206 _]
          tunnel: w927 -> [w1205 _]
          tunnel: [w1206 w1207] -> w916
          tunnel: [w1205 w1208] -> w814
          tunnel: "goniometer PWM\n offset" -> [_ w1208]
          tunnel: "delta PWM offset" -> [_ w1207]
          frame False {
          }
          frame True {
          }
        }
        n255 = Index Array(array=w805, index (row)=w881, index (col)=w881) -> (element=w804:dbl)
        n256 = Index Array(array=w806, index (row)=w880, index (col)=w880) -> (element=w801:dbl)
        n257 = local read "SynPulseOn"() -> (w759:bool)
        n258 = local read "Straight"() -> (w744:bool)
        n259 = To Double Precision Float(number=w754) -> (double precision float=w894:dbl)
        n260 = Index Array(array=w806, index (row)=w808, index (col)=w808) -> (element=w800:dbl)
        n261 = Index Array(array=w805, index (row)=w810, index (col)=w810) -> (element=w803:dbl)
        n262 = local read "op-space pos\n(global frame)"() -> (w952:dbl[])
        n263 = local read "changes from \nadmittance {m}"() -> (w951:dbl[])
        n264 = Index Array(array=w806, index (row)=w807, index (col)=w807) -> (element=w799:dbl)
        n265 = Index Array(array=w805, index (row)=w809, index (col)=w809) -> (element=w802:dbl)
        n266 = local read "Mouse forces"() -> (w904:dbl[])
        n267 = local read "Joint_pos (rad)"() -> (w953:dbl[])
        n268 = Build Array(w804, w803, w802) -> (w798:dbl[])
        n269 = Build Array(w801, w800, w799) -> (w797:dbl[])
        n270 = Build Array(FALSE ("element"), FALSE ("element"), w744, w759) -> (w782:bool[])
        n271 = Boolean To (0,1)(Boolean=w782) -> (0, 1=w781:i16[])
        n272 = To Double Precision Float(number=w781) -> (double precision float=w780:dbl[])
        n273 = Build Array (concatenate)(w953, w952, w951, w894, w916, w814, w904, w798, w797, w780) -> (w950:dbl[])
        n274 = Index Array(array=w916, index=1) -> (element=w816:dbl)
        n275 = Index Array(array=w916, index=2) -> (element=w815:dbl)
        n276 = Index Array(array=w916, index=0) -> (element=w817:dbl)
        n277 = Decimate 1D Array(w950) -> (w949:dbl[], w948:dbl[], w947:dbl[], w946:dbl[], w945:dbl[], w944:dbl[], w943:dbl[], w942:dbl[], w941:dbl[], w940:dbl[], w939:dbl[], w938:dbl[], w937:dbl[], w936:dbl[], w935:dbl[], w934:dbl[], w933:dbl[], w932:dbl[], w931:dbl[], w843:dbl[], w842:dbl[], w841:dbl[], w840:dbl[], w796:dbl[], w795:dbl[], w794:dbl[], w793:dbl[], w779:dbl[], w778:dbl[], w777:dbl[], w758:dbl[])
        n278 = In Range and Coerce(upper limit=99.0, x=w817, lower limit=1.0) -> (coerced(x)=w821:dbl)  [unwired: 1 out]
        n279 = In Range and Coerce(upper limit=99.0, x=w816, lower limit=1.0) -> (coerced(x)=w820:dbl)  [unwired: 1 out]
        n280 = In Range and Coerce(upper limit=99.0, x=w815, lower limit=1.0) -> (coerced(x)=w819:dbl)  [unwired: 1 out]
        n281 = In Range and Coerce(upper limit=99.0, x=w814, lower limit=1.0) -> (coerced(x)=w818:dbl)  [unwired: 1 out]
        n282 = Build Array(w949, w948, w947, w946, w945, w944, w943, w942, w941, w940, w939, w938, w937, w936, w935, w934, w933, w932, w931, w843, w842, w841, w840, w796, w795, w794, w793, w779, w778, w777, w758) -> (→"Data output":dbl[][])
        n283 = Tick Count (ms)() -> (millisecond timer value=w924:u32)
        n284 = shared-variable "RT CompactRIO Target\\Mod5\\PWM2"(w819) -> ()  [unwired: 1 in, 1 out]
        n285 = shared-variable "RT CompactRIO Target\\Mod5\\PWM0"(w821) -> ()  [unwired: 1 in, 1 out]
        n286 = Subtract(x=w924, y=w923) -> (x-y=→"True loop time (ms)":u32)
        n287 = shared-variable "RT CompactRIO Target\\Mod5\\PWM1"(w820) -> ()  [unwired: 1 in, 1 out]
        n288 = shared-variable "RT CompactRIO Target\\Mod5\\PWM3"(w818) -> ()  [unwired: 1 in, 1 out]
        n289 = disable-structure shown="Enabled" {
          disable-tunnel: w916 -> [w1029 _]
          disable-tunnel: w814 -> [w1028 _]
          frame Enabled {
            n290 = local read "changes from \nadmittance {m}"() -> (w1031:dbl[])
            n291 = local read "Mouse forces"() -> (w1030:dbl[])
            n292 = local read "op-space pos\n(global frame)"() -> (w1053:dbl[])
            n293 = Array Subset(array=w1031, index=0, length=3) -> (w1039:dbl[])
            n294 = Array Subset(array=w1031, index=3, length=1) -> (w1034:dbl[])
            n295 = Build Array (concatenate)(w1029, w1028) -> (w1051:dbl[])
            n296 = Array Subset(array=w1030, index=0, length=3) -> (w1047:dbl[])
            n297 = Array Subset(array=w1030, index=3, length=1) -> (w1042:dbl[])
            n298 = Array To Cluster(array=w1053) -> (cluster=→"XY position" →"Z position" →"alpha beta gamma":T8)
            n299 = Array To Cluster(array=w1034) -> (cluster=→"Admittance changes in Yaw":T4)
            n300 = Array To Cluster(array=w1039) -> (cluster=→"Admittance changes in XY":T4)
            n301 = Reshape Array(w1051, 4 ("dimension size")) -> (w1049:dbl[])
            n302 = Array To Cluster(array=w1042) -> (cluster=→"Torques (Nm)":T4)
            n303 = Array To Cluster(array=w1047) -> (cluster=→"Forces (N)":T4)
            n304 = Array To Cluster(array=w1049) -> (cluster=→"PWM":T4)
          }
          frame Disabled {
          }
        }
        n305 = node-c288() -> ()  [unwired: 1 in, 1 out]
        "loop" <- w882
        "m_applied" <- "m"
        "c_applied" <- "c"
        "Mousetrack ON" <- "Mousetrack on"
      }
      n306 = node-c288(w728) -> ()  [unwired: 1 out]
    }
    frame #6 {
      n307 = while "Joint space control" {
        stop <- FALSE stop-if-true
        n308 = local read "Joint_pos (rad)"() -> (w1230:dbl[])
        n309 = local read "theta1,2,3"() -> (w1235:dbl)
        n310 = local read "theta6"() -> (w1234:dbl)
        n311 = Build Array(w1235, w1235, w1235, w1234) -> (w1243:dbl[])
        n312 = local read "Theta output range"() -> (w1231:cluster{"output high":dbl, "output low":dbl}[])
        n313 = local read "Theta PID gains"() -> (w1232:T2)
        n314 = call-poly <vilib>:"PID.vi"("output range"=w1231, "PID gains"=w1232, "process variable"=w1230, "setpoint"=w1243) -> ("output"=w1238:dbl[])  [unwired: 6 in, 1 out]
        n315 = Add(x=w1238, y=dbl[] [50.0, 50.0, 50.0, 50.0]) -> (x+y=w1236:dbl[])
        n316 = Index Array(array=w1236, index=0) -> (element=w1217:dbl)
        n317 = Index Array(array=w1236, index=1) -> (element=w1216:dbl)
        n318 = Index Array(array=w1236, index=2) -> (element=w1215:dbl)
        n319 = Index Array(array=w1236, index=3) -> (element=w1214:dbl)
        n320 = In Range and Coerce(upper limit=99.0, x=w1217, lower limit=1.0) -> (coerced(x)=w1221:dbl)  [unwired: 1 out]
        n321 = In Range and Coerce(upper limit=99.0, x=w1216, lower limit=1.0) -> (coerced(x)=w1220:dbl)  [unwired: 1 out]
        n322 = In Range and Coerce(upper limit=99.0, x=w1215, lower limit=1.0) -> (coerced(x)=w1219:dbl)  [unwired: 1 out]
        n323 = In Range and Coerce(upper limit=99.0, x=w1214, lower limit=1.0) -> (coerced(x)=w1218:dbl)  [unwired: 1 out]
        n324 = shared-variable "RT CompactRIO Target\\Mod5\\PWM0"(w1221) -> ()  [unwired: 1 in, 1 out]
        n325 = shared-variable "RT CompactRIO Target\\Mod5\\PWM2"(w1219) -> ()  [unwired: 1 in, 1 out]
        n326 = shared-variable "RT CompactRIO Target\\Mod5\\PWM1"(w1220) -> ()  [unwired: 1 in, 1 out]
        n327 = shared-variable "RT CompactRIO Target\\Mod5\\PWM3"(w1218) -> ()  [unwired: 1 in, 1 out]
      }
      n328 = local write "Record to current file"(FALSE ("Record to current file")) -> ()
    }
  }
  n329 = node-c288(i64 2 ("Period")) -> (w4:T5)  [unwired: 3 in]
  n330 = while "Avoid Delta robot joint collision with platform" {
    stop <- FALSE stop-if-true
    n331 = local read "Joint_pos (rad)"() -> (w1250:dbl[])
    n332 = Wait (ms)(milliseconds to wait=u32 25) -> ()  [unwired: 1 out]
    n333 = Array Subset(array=w1250, index=0, length=3) -> (w1247:dbl[])
    n334 = Less?(x=w1247, y=dbl[] [-0.85, -0.85, -0.85]) -> (x < y?=w1252:bool[])
    n335 = Or Array Elements(Boolean array=w1252) -> (logical OR=w1244:bool)
    n336 = local write "Out of range"(w1244) -> ()
  }
  n337 = while "Encoder counts to Joint position" {
    stop <- FALSE stop-if-true
    n338 = local read "Loop time (ms)"() -> (w1265:i64)
    n339 = call "cRIO_4DoF_Encoders_counts2rad(subVI).vi"() -> ("Theta3"=w1260:dbl, "Theta2"=w1261:dbl, "Theta1"=w1262:dbl, "Theta6"=w1266:dbl)  [unwired: 4 in]
    n340 = Build Array(w1262, w1261, w1260, w1266) -> (w1259:dbl[])
    n341 = Divide "offset"(x=3.141592653589793, y=4.0) -> (x/y=w1258:dbl)
    n342 = Wait (ms)(milliseconds to wait=w1265) -> ()  [unwired: 1 out]
    n343 = Build Array(w1258, w1258, w1258, 0.0 ("element")) -> (w1256:dbl[])
    n344 = Subtract(x=w1259, y=w1256) -> (x-y=w1255:dbl[])
    n345 = Subtract(x=w1255, y="Joint offset") -> (x-y=→"Joint_pos (rad)":dbl[])
  }
  n346 = timed-loop {
    timing: w4 -> [_]
    timing-out: [_] -> w3
    stop <- FALSE stop-if-true
    n347 = node-c288() -> ()  [unwired: 1 in, 1 out]
    n348 = local read "Sensor V offset"() -> (w1271:dbl[])
    n349 = call "cRIO_4DoF_Fsample.vi"("Sensor V offset"=w1271) -> ("F"=→"F":dbl[], "Array"=→"Raw voltages":dbl[])  [unwired: 9 in]
    n350 = node-c288() -> ()  [unwired: 1 in, 1 out]
  }
  n351 = node-c288(w3) -> ()  [unwired: 1 out]
  n352 = while "Force sensor voltages to Forces and torques" {
    stop <- FALSE stop-if-true
    n353 = local read "Loop time (ms)"() -> (w1279:i64)
    n354 = Wait (ms)(milliseconds to wait=w1279) -> ()  [unwired: 1 out]
    n355 = flat-sequence {
      tunnel: [w1288] -> w1276
      tunnel: "number Fsamples" -> [w1287]
      tunnel: w1276 -> [w1294]
      tunnel: [w1293] -> w1275
      frame #0 {
        n356 = for {
          N: w1287 -> [_]
          tunnel: [w1291] -> w1289 mode=indexing
          n357 = Wait (ms)(milliseconds to wait=u32 1) -> ()  [unwired: 1 out]
          n358 = local read "F"() -> (w1291:dbl[])
        }
        n359 = Transpose 2D Array(2D array=w1289) -> (transposed array=w1288:dbl[][])
      }
      frame #1 {
        n360 = for {
          N: 4 -> [_]
          tunnel: w1294 -> [w1296] mode=indexing
          tunnel: [w1295] -> w1293 mode=indexing
          n361 = call-poly <vilib>:"Mean.vi"("X"=w1296) -> ("mean"=w1295:dbl)  [unwired: 1 out]
        }
      }
    }
    n362 = Array Subset(array=w1275, index=0, length=3) -> (w1278:dbl[])
    n363 = Array Subset(array=w1275, index=3, length=1) -> (w1277:dbl[])
    n364 = global write "Global 1.vi" "F_measured"(w1275) -> ()
    n365 = Array To Cluster(array=w1278) -> (cluster=→"Forces (N) 2":T4)
    n366 = Array To Cluster(array=w1277) -> (cluster=→"Torques (Nm) 2":T4)
    "F_measured" <- w1275
  }
  n367 = while "Data saving loop... a new file needs to be created for each data set using the \"Write data to file (PC VI).vi\"" {
    stop <- FALSE stop-if-true
    n368 = flat-sequence "Data Saving" {
      tunnel: [w1311] -> w1304
      tunnel: [w1312] -> w1303
      tunnel: w1304 -> [w1314]
      tunnel: [w1314] -> w1300
      tunnel: w1303 -> [w1313]
      tunnel: [w1313] -> w1298
      tunnel: w1300 -> [w1320]
      tunnel: [w1320] -> w1299
      tunnel: w1298 -> [w1319]
      tunnel: [w1319] -> w1297
      tunnel: w1299 -> [w1322]
      tunnel: w1297 -> [w1323]
      tunnel: [w1321] -> w1302
      tunnel: w1302 -> [w1341]
      frame #0 {
        # "Open network stream endpoint"
        n369 = local write "Data syncing"(FALSE ("Activate")) -> ()
        n370 = Create Network Stream Writer Endpoint(7:1000 ("writer buffer size"), 9:dbl[][] [] ("appended array"), 11:"cRIO_Write_Data" ("writer name")) -> (0:w1309:errorcluster, 3:w1310:refnum<k21>)  [unwired: 4 in]
        n371 = Flush Stream(8:w1309, 11:w1310) -> (0:w1311:errorcluster, 3:w1312:refnum<k21>)  [unwired: 2 in, 1 out]
      }
      frame #1 {
        # "Begin Saving Data"
        n372 = while {
          stop <- "BEGIN saving new data set" stop-if-true
          n373 = Wait (ms)(milliseconds to wait=u32 250) -> ()  [unwired: 1 out]
        }
      }
      frame #2 {
        # "Start Pulse Sync loop"
        n374 = local write "Data syncing"(TRUE) -> ()
        n375 = Wait (ms)(milliseconds to wait=u32 250) -> ()  [unwired: 1 out]
      }
      frame #3 {
        # "Save Data by writing elements to network stream -/-/-/-/ and Pause Saving if necessary, by increasing loop time"
        n376 = while {
          tunnel: w1323 -> [w1331]
          tunnel: w1322 -> [w1330]
          tunnel: [w1326] -> w1321
          stop <- "STOP saving data set" stop-if-true
          n377 = local read "Data output"() -> (w1325:dbl[][])
          n378 = local write "Data syncing"(TRUE ("Data syncing")) -> ()
          n379 = shared-variable-write "Write Single Element to Stream"(w1331, w1330, w1325) -> (w1334:refnum<k21>, →"network stream":errorcluster)  [unwired: 1 in, 1 out]
          n380 = property class="Network Stream Endpoint"(reference=w1334) -> (reference out=w1326:refnum<k21>, "AvailElmntsForWrite"=→"Available Elements for Writing in network stream":i32)  [unwired: 1 in, 1 out]
          n381 = case shown="False" "PAUSE saving data set" {
            tunnel: [w1335 "PAUSE ms to wait"] -> w1327
            frame False {
              n382 = local read "Loop time (ms)"() -> (w1335:i64)
            }
            frame True {
            }
          }
          n383 = Wait (ms)(milliseconds to wait=w1327) -> ()  [unwired: 1 out]
        }
      }
      frame #4 {
        # "Stop"
        n384 = Flush Stream(11:w1341) -> (3:w1342:refnum<k21>)  [unwired: 3 in, 2 out]
        n385 = local write "BEGIN saving new data set"(FALSE ("BEGIN SAVING DATA")) -> ()
        n386 = local write "Data syncing"(FALSE ("Data syncing")) -> ()
        n387 = local write "STOP saving data set"(FALSE ("STOP SAVING DATA")) -> ()
        n388 = local write "PAUSE saving data set"(FALSE ("PAUSE SAVING DATA")) -> ()
        n389 = Destroy Stream Endpoint(11:w1342) -> ()  [unwired: 1 in, 1 out]
      }
    }
  }
  n390 = while {
    shift-right: [w1349] -> _
    shift-left: _ -> [w1350]
    shift-right: [w1346] -> _
    shift-left: i16 0 -> [w1345]
    stop <- FALSE stop-if-true
    n391 = local read "op-space pos\n(global frame)"() -> (w1368:dbl[])
    n392 = Add(x="Rentry", y="Loop radius") -> (x+y=w1343:dbl)
    n393 = Negate(x=w1343) -> (-x=w1344:dbl)
    n394 = Negate(x="Rentry") -> (-x=w1355:dbl)
    n395 = Build Array("Rentry", w1344) -> (→"entry_cen":dbl[])
    n396 = Build Array(w1355, w1344) -> (→"exit_cen":dbl[])
    n397 = Index Array(array=w1368, index=0) -> (element=w1360:dbl)
    n398 = Add(x="Loop offset", y=0.001) -> (x+y=w1358:dbl)
    n399 = Negate(x=w1358) -> (-x=w1367:dbl)
    n400 = In Range and Coerce(upper limit=w1358, x=w1360, lower limit=w1367) -> (In Range?=w1351:bool)  [unwired: 1 out]
    "Straight" <- w1351
    n401 = Not(x=w1351) -> (.not. x?=w1361:bool)
    n402 = Greater?(x=w1360, y=0.0) -> (0:w1365:bool)
    n403 = And(x=w1365, y=w1361) -> (x .and. y?=→"Loop_R":bool)
    n404 = local read "Loop time (ms)"() -> (w1369:i64)
    n405 = Less?(x=w1360, y=0.0) -> (x < y?=w1362:bool)
    n406 = Wait (ms)(milliseconds to wait=w1369) -> ()  [unwired: 1 out]
    n407 = And(x=w1362, y=w1361) -> (x .and. y?=w1349:bool)
    "Loop_L" <- w1349
    n408 = Greater?(x=w1349, y=w1350) -> (0:w1348:bool)
    n409 = Boolean To (0,1)(Boolean=w1348) -> (0, 1=w1347:i16)
    n410 = Add(x=w1347, y=w1345) -> (x+y=w1346:i16)
    "Number of laps" <- w1346
    "Rexit" <- "Rentry"
  }
  n411 = while "Measure force sensor voltage offset" {
    shift-right: [w1380] -> _
    shift-left: _ -> [w1379]
    i -> [w1376]
    stop <- FALSE stop-if-true
    n412 = Wait (ms)(milliseconds to wait=u32 250) -> ()  [unwired: 1 out]
    n413 = Less?(x=w1376, y=2) -> (x < y?=w1374:bool)
    n414 = Or(x="Measure Fsensor \nV offset", y=w1374) -> (x .or. y?=w1373:bool)
    n415 = case shown="True" w1373 {
      tunnel: [w1381 w1383] -> w1380
      tunnel: w1379 -> [w1381 _]
      frame False {
      }
      frame True {
        n416 = flat-sequence {
          tunnel: [w1385] -> w1384
          tunnel: w1384 -> [w1391]
          tunnel: [w1390] -> w1382
          tunnel: [w1396] -> w1383
          tunnel: w1382 -> [w1396]
          frame #0 {
            n417 = for {
              N: 20 -> [_]
              tunnel: [w1389] -> w1386 mode=indexing
              n418 = local read "Raw voltages"() -> (w1389:dbl[])
              n419 = Wait (ms)(milliseconds to wait=u32 1) -> ()  [unwired: 1 out]
            }
            n420 = Transpose 2D Array(2D array=w1386) -> (transposed array=w1385:dbl[][])
          }
          frame #1 {
            n421 = for {
              N: 6 -> [_]
              tunnel: w1391 -> [w1394] mode=indexing
              tunnel: [w1393] -> w1390 mode=indexing
              n422 = call-poly <vilib>:"Mean.vi"("X"=w1394) -> ("mean"=w1393:dbl)  [unwired: 1 out]
            }
          }
          frame #2 {
            n423 = local write "Measure Fsensor \nV offset"(FALSE ("DAQ V offset")) -> ()
          }
        }
      }
    }
    "Sensor V offset" <- w1380
  }
  n424 = while {
    stop <- FALSE stop-if-true
    n425 = flat-sequence {
      frame #0 {
        n426 = while {
          shift-right: [w1400] -> _
          shift-left: _ -> [w1399]
          stop <- w1400 stop-if-true
          n427 = local read "Mousetrack on"() -> (w1400:bool)
          n428 = Wait (ms)(milliseconds to wait=u32 10) -> ()  [unwired: 1 out]
          n429 = Greater?(x=w1400, y=w1399) -> (0:w1398:bool)
          n430 = case shown="True" w1398 {
            frame False {
            }
            frame True {
              n431 = local write "delpos limits (+/-)\nadmittance control \n(mouse frame)"(dbl[] [0.0012, 0.0002, 0.0, 0.01] ("delpos limits (+/-)\nadmittance control \nDzone")) -> ()
            }
          }
          n432 = case shown="True" w1400 {
            frame False {
              n433 = for {
                N: 1 -> [_]
                w1405 = FALSE
                n434 = Wait (ms)(milliseconds to wait=u32 100) -> ()  [unwired: 1 out]
                n435 = local write "Y_trajectory"(w1405) -> ()
                n436 = local write "Yaw_tajectory"(w1405) -> ()
              }
            }
            frame True {
              n437 = local write "Yaw_tajectory"(TRUE ("Mousetrack_Y")) -> ()
              n438 = local write "Y_trajectory"(TRUE ("Mousetrack_Y")) -> ()
            }
          }
        }
      }
      frame #1 {
        n439 = local read "op-space pos\n(global frame)"() -> (w1410:dbl[])
        n440 = Index Array(array=w1410, index=3) -> (element=w1408:dbl)
        n441 = while {
          tunnel: w1408 -> [w1415]
          stop <- w1420 stop-if-true
          n442 = local read "Straight"() -> (w1412:bool)
          n443 = local read "Loop radius"() -> (w1413:dbl)
          n444 = local read "op-space pos\n(global frame)"() -> (w1416:dbl[])
          n445 = mathscript code="xpos = Pos(1,1);\nypos = Pos(1,2);\nzpos = Pos(1,3);\nyawpos = Pos(1,4);\n\n% round to nearest pi\nyawtarg = real(round((yaw_init /pi))*pi );\n\nif all(Straight)\n    if ypos > 0 \n        ytarg = R;\n    else\n        ytarg = -R;        \n    end\nelse\n    ytarg = ypos;\nend\n\ntargetpos = [xpos, ytarg, zpos, yawtarg];\n\ndelpos = real(targetpos - Pos);"("Pos"=w1416, "yaw_init"=w1415, "R"=w1413, "Straight"=w1412) -> ("delpos"=w1411:dbl[])  [unwired: 1 in, 1 out]
          n446 = local read "Straight"() -> (w1423:bool)
          n447 = local read "Loop_R"() -> (w1418:bool)
          n448 = local read "Mousetrack on"() -> (w1422:bool)
          n449 = local read "Loop_L"() -> (w1419:bool)
          n450 = Or(x=w1419, y=w1418) -> (x .or. y?=w1417:bool)
          n451 = Not(x=w1423) -> (.not. x?=w1425:bool)
          n452 = local read "Loop time (ms)"() -> (w1414:i64)
          n453 = Not(x=w1422) -> (.not. x?=w1421:bool)
          n454 = local write "deltapos"(w1411) -> ()
          n455 = And(x=w1425, y=w1417) -> (x .and. y?=w1424:bool)
          n456 = Or(x=w1424, y=w1421) -> (x .or. y?=w1420:bool)
          n457 = Wait (ms)(milliseconds to wait=w1414) -> ()  [unwired: 1 out]
        }
      }
      frame #2 {
        n458 = while {
          stop <- w1626 stop-if-true
          n459 = local read "op-space pos\n(global frame)"() -> (w1622:dbl[])
          n460 = local read "Loop radius"() -> (w1620:dbl)
          n461 = local read "Loop offset"() -> (w1611:dbl)
          n462 = mathscript code="Rcen = Ofst;     % center of right loop = (Ofst,0)\nLcen = -Ofst;     % center of left loop = (-Ofst,0)\nxpos = Pos(1,1);\nypos = Pos(1,2);\nzpos = Pos(1,3);\nyawpos = Pos(1,4);\n\nRotz = [cos(yawpos),-sin(yawpos),0; sin(yawpos),cos(yawpos),0; 0,0,1];\nxhat = [1, 0, 0]';\nzhat = [0, 0, 1]';\n\nif xpos > 0    % right loop\n       xcen = xpos - Rcen;\n       ycen = ypos;\n       Rmag = real((xcen^2 + ycen^2)^0.5);\n       xtarg = R/Rmag*xcen  + Rcen;\n       ytarg = R/Rmag*ycen;      \n       RLsgn = -1;  % anti clockwise\nelse % left loop\n       xcen = xpos - Lcen;\n       ycen = ypos;\n       Rmag = real((xcen^2 + ycen^2)^0.5);\n       xtarg = R/Rmag*xcen + Lcen;\n       ytarg = R/Rmag*ycen; \n       RLsgn = -1;    \nend\n\nvecpos = [xcen, ycen, 0]';         % position vector, zero'd circle\nvecyaw = RLsgn*cross(vecpos,zhat);  % yaw vector\nvecyaw_o = Rotz'*vecyaw;        %  yaw vector transformed by actual yaw\nyawerrsign = sign(0 - vecyaw_o(2));  % sign of yaw error\nyawerrmag = acos(dot(vecyaw_o,xhat)/(norm(vecyaw_o)*norm(xhat))); % magnitude of yaw error   \nyawtarg  = yawpos - yawerrsign*real(yawerrmag); % target yaw position\n\ntargetpos = [xtarg, ytarg, zpos, yawtarg];\n\ndelpos = real(targetpos - Pos);"("Pos"=w1622, "R"=w1620, "Ofst"=w1611) -> ("delpos"=w1619:dbl[], "Rotz"=→"Rotz":dbl[][], "targetpos"=→"targetpos":dbl[], "Pos"=→"Pos":dbl[])  [unwired: 1 in, 1 out]
          n463 = local read "Straight"() -> (w1616:bool)
          n464 = local read "Loop_L"() -> (w1623:bool)
          n465 = local read "Loop_R"() -> (w1624:bool)
          n466 = local read "Mousetrack on"() -> (w1625:bool)
          n467 = local read "Loop time (ms)"() -> (w1621:i64)
          n468 = Or(x=w1623, y=w1624) -> (x .or. y?=w1618:bool)
          n469 = Not(x=w1618) -> (.not. x?=w1617:bool)
          n470 = local write "deltapos"(w1619) -> ()
          n471 = Not(x=w1625) -> (.not. x?=w1627:bool)
          n472 = Or(x=w1616, y=w1617) -> (x .or. y?=w1615:bool)
          n473 = Or(x=w1615, y=w1627) -> (x .or. y?=w1626:bool)
          n474 = Wait (ms)(milliseconds to wait=w1621) -> ()  [unwired: 1 out]
        }
      }
    }
  }
  n475 = while {
    shift-right: ["Joystick control on"] -> _
    shift-left: _ -> [w2085]
    shift-right: [w2078] -> _
    shift-left: _ -> [w2079]
    i -> [w2082]
    stop <- FALSE stop-if-true
    n476 = shared-variable "RT CompactRIO Target\\Mod8\\AI29"() -> (w2088:dbl)  [unwired: 1 in, 1 out]
    n477 = shared-variable "RT CompactRIO Target\\Mod8\\AI23"() -> (w2086:dbl)  [unwired: 1 in, 1 out]
    n478 = shared-variable "RT CompactRIO Target\\Mod8\\AI21"() -> (w2091:dbl)  [unwired: 1 in, 1 out]
    n479 = shared-variable "RT CompactRIO Target\\Mod8\\AI22"() -> (w2090:dbl)  [unwired: 1 in, 1 out]
    n480 = shared-variable "RT CompactRIO Target\\Mod8\\AI30"() -> (w2087:dbl)  [unwired: 1 in, 1 out]
    n481 = shared-variable "RT CompactRIO Target\\Mod8\\AI31"() -> (w2089:dbl)  [unwired: 1 in, 1 out]
    n482 = Less?(x=w2082, y=2) -> (x < y?=w2080:bool)
    n483 = Build Array(w2091, w2090, w2088, w2087, w2086, w2089) -> (w2084:dbl[])
    "Joystick input" <- w2084
    n484 = case shown="True" w2080 {
      tunnel: [w2100 w2101] -> w2078
      tunnel: w2079 -> [w2100 _]
      frame False {
      }
      frame True {
        n485 = flat-sequence {
          tunnel: [w2103] -> w2102
          tunnel: w2102 -> [w2112]
          tunnel: [w2111] -> w2101
          frame #0 {
            n486 = for {
              N: 20 -> [_]
              tunnel: [w2106] -> w2104 mode=indexing
              n487 = shared-variable "RT CompactRIO Target\\Mod8\\AI29"() -> (w2108:dbl)  [unwired: 1 in, 1 out]
              n488 = shared-variable "RT CompactRIO Target\\Mod8\\AI21"() -> (w2110:dbl)  [unwired: 1 in, 1 out]
              n489 = shared-variable "RT CompactRIO Target\\Mod8\\AI22"() -> (w2109:dbl)  [unwired: 1 in, 1 out]
              n490 = shared-variable "RT CompactRIO Target\\Mod8\\AI30"() -> (w2107:dbl)  [unwired: 1 in, 1 out]
              n491 = Build Array(w2110, w2109, w2108, w2107) -> (w2106:dbl[])
            }
            n492 = Transpose 2D Array(2D array=w2104) -> (transposed array=w2103:dbl[][])
          }
          frame #1 {
            n493 = for {
              N: 4 -> [_]
              tunnel: w2112 -> [w2115] mode=indexing
              tunnel: [w2114] -> w2111 mode=indexing
              n494 = call-poly <vilib>:"Mean.vi"("X"=w2115) -> ("mean"=w2114:dbl)  [unwired: 1 out]
            }
          }
        }
      }
    }
    "Jostick offset" <- w2078
    n495 = Array Subset(array=w2084, index=0, length=4) -> (w2096:dbl[])
    n496 = Subtract(x=w2096, y=w2078) -> (x-y=w2095:dbl[])
    n497 = Multiply(x=w2095, y=dbl[] [0.4, 0.4, 0.0, 0.04]) -> (x*y=w2093:dbl[])
    n498 = case shown="False" "Joystick control on" {
      selector: "Joystick control on" -> [w2119 _]
      tunnel: w2093 -> [_ w2122]
      tunnel: w2085 -> [w2118 _]
      frame False {
        n499 = Greater?(x=w2118, y=w2119) -> (0:w2120:bool)
        n500 = case shown="False" w2120 {
          frame False {
          }
          frame True {
            n501 = local write "Manual forces\n(mouse frame)"(dbl[] [0.0, 0.0, 0.0, 0.0]) -> ()
          }
        }
      }
      frame True {
        n502 = local write "Manual forces\n(mouse frame)"(w2122) -> ()
      }
    }
    n503 = case shown="False" "Joystick control on" {
      tunnel: [u32 100 ("Loop time (ms) FDAQ") w2117] -> w2092
      frame False {
      }
      frame True {
        n504 = local read "Loop time (ms)"() -> (w2117:i64)
      }
    }
    n505 = Wait (ms)(milliseconds to wait=w2092) -> ()  [unwired: 1 out]
  }
  n506 = while {
    stop <- FALSE stop-if-true
    n507 = flat-sequence {
      frame #0 {
        n508 = while {
          i -> [w2124]
          stop <- w2127 stop-if-true
          n509 = flat-sequence {
            frame #0 {
              n510 = case shown="False" "Manual \npulse low" {
                tunnel: [TRUE ("DIO0") FALSE ("DIO0")] -> w2130
                frame False {
                }
                frame True {
                }
              }
              n511 = Wait (ms)(milliseconds to wait=u32 100) -> ()  [unwired: 1 out]
              n512 = local write "SynPulseOn"(w2130) -> ()
              n513 = shared-variable "RT CompactRIO Target\\Mod7\\DIO0"(w2130) -> ()  [unwired: 1 in, 1 out]
            }
            frame #1 {
              n514 = case shown="True" "Manual \npulse high" {
                tunnel: [FALSE ("DIO0") TRUE ("DIO0")] -> w2135
                frame False {
                }
                frame True {
                }
              }
              n515 = shared-variable "RT CompactRIO Target\\Mod7\\DIO0"(w2135) -> ()  [unwired: 1 in, 1 out]
              n516 = local write "SynPulseOn"(w2135) -> ()
              n517 = Wait (ms)(milliseconds to wait=u32 900) -> ()  [unwired: 1 out]
            }
          }
          n518 = local read "Data syncing"() -> (w2128:bool)
          n519 = local read "STOP saving data set"() -> (w2126:bool)
          n520 = Not(x=w2128) -> (.not. x?=w2125:bool)
          n521 = Or(x=w2125, y=w2126) -> (x .or. y?=w2127:bool)
          "Sync_pulse" <- w2124
        }
      }
    }
  }
  n522 = while {
    stop <- FALSE stop-if-true
    n523 = flat-sequence {
      tunnel: [w2164] -> w2139
      tunnel: w2139 -> [w2591]
      frame #0 {
        n524 = local write "End Wheel"(FALSE ("End Wheel")) -> ()
        n525 = Wait (ms)(milliseconds to wait=u32 250) -> ()  [unwired: 1 out]
      }
      frame #1 {
        n526 = while {
          stop <- w2143 stop-if-true
          n527 = local read "End Wheel"() -> (w2143:bool)
          n528 = Wait (ms)(milliseconds to wait=u32 250) -> ()  [unwired: 1 out]
        }
      }
      frame #2 {
        n529 = while {
          shift-right: [w2147] -> _
          shift-left: TRUE -> [w2148]
          stop <- w2160 stop-if-true
          n530 = local read "op-space pos\n(global frame)"() -> (w2155:dbl[])
          n531 = Wait (ms)(milliseconds to wait=u32 10) -> ()  [unwired: 1 out]
          n532 = local read "exit_cen"() -> (w2153:dbl[])
          n533 = Index Array(array=w2155, index=0) -> (element=w2154:dbl)
          n534 = Index Array(array=w2153, index=0) -> (element=w2151:dbl)
          n535 = Index Array(array=w2155, index=1) -> (element=w2158:dbl)
          n536 = local read "Straight"() -> (w2149:bool)
          n537 = Greater?(x=w2154, y=w2151) -> (0:w2147:bool)
          n538 = Less?(x=w2158, y=0.0) -> (x < y?=w2150:bool)
          n539 = Greater?(x=w2147, y=w2148) -> (0:w2146:bool)
          n540 = Compound Arithmetic op=AND(w2149, w2150, w2146) -> (w2160:bool)
        }
      }
      frame #3 {
        n541 = local write "delpos limits (+/-)\nadmittance control \n(mouse frame)"(dbl[] [0.0008, 0.0, 0.0, 0.0] ("delpos limits (+/-)\nadmittance control \nDzone")) -> ()
        n542 = local write "Mousetrack on"(FALSE ("Eight maze on")) -> ()
      }
      frame #4 {
        n543 = while {
          tunnel: [w2168] -> w2164
          stop <- w2170 stop-if-true
          n544 = local read "exit_cen"() -> (w2165:dbl[])
          n545 = local read "Rexit"() -> (w2177:dbl)
          n546 = local read "op-space pos\n(global frame)"() -> (w2168:dbl[])
          n547 = mathscript code="xpos = Pos(1,1);\nypos = Pos(1,2);\nzpos = Pos(1,3);\nyawpos = Pos(1,4);\n\nRotz = [cos(yawpos),-sin(yawpos),0; sin(yawpos),cos(yawpos),0; 0,0,1];\nxhat = [1, 0, 0]';\nzhat = [0, 0, 1]';\n\nRLsgn = 1; % clockwise\n\nxcen = xpos - w_cen(1);\nycen = ypos - w_cen(2);\nRmag = real((xcen^2 + ycen^2)^0.5);\nxtarg = R/Rmag*xcen  + w_cen(1);\nytarg = R/Rmag*ycen + w_cen(2);      \n\nvecpos = [xcen, ycen, 0]';         % position vector, zero'd circle\nvecyaw = RLsgn*cross(vecpos,zhat);  % yaw vector\nvecyaw_o = Rotz'*vecyaw;        %  yaw vector transformed by actual yaw\nyawerrsign = sign(0 - vecyaw_o(2));  % sign of yaw error\nyawerrmag = acos(dot(vecyaw_o,xhat)/(norm(vecyaw_o)*norm(xhat))); % magnitude of yaw error   \nyawtarg  = yawpos - yawerrsign*real(yawerrmag); % target yaw position\n\ntargetpos = [xtarg, ytarg, zpos, yawtarg];\n\ndelpos = real(targetpos - Pos);"("Pos"=w2168, "R"=w2177, "w_cen"=w2165) -> ("delpos"=w2169:dbl[], "Rmag"=→"Rmag":dbl)  [unwired: 1 in, 1 out]
          n548 = local read "op-space pos\n(global frame)"() -> (w2176:dbl[])
          n549 = local read "exit_cen"() -> (w2172:dbl[])
          n550 = Index Array(array=w2176, index=1) -> (element=w2174:dbl)
          n551 = Index Array(array=w2172, index=1) -> (element=w2171:dbl)
          n552 = Less?(x=w2174, y=w2171) -> (x < y?=w2170:bool)
          n553 = local write "deltapos"(w2169) -> ()
          n554 = Wait (ms)(milliseconds to wait=u32 10) -> ()  [unwired: 1 out]
        }
      }
      frame #5 {
        n555 = while {
          tunnel: w2591 -> [w2600]
          stop <- w2593 stop-if-true
          n556 = local read "op-space pos\n(global frame)"() -> (w2596:dbl[])
          n557 = local read "op-space pos\n(global frame)"() -> (w2599:dbl[])
          n558 = Index Array(array=w2596, index=1) -> (element=w2595:dbl)
          n559 = Index Array(array=w2600, index=3) -> (element=w2601:dbl)
          n560 = mathscript code="xpos = Pos(1,1);\nypos = Pos(1,2);\nzpos = Pos(1,3);\nyawpos = Pos(1,4);\n\nyawtarg = real(round((yaw_init)/(pi/2))*pi/2);\n\nxtarg = 0;\n\ntargetpos = [xtarg, ypos, zpos, yawtarg];\n\ndelpos = real(targetpos - Pos);"("yaw_init"=w2601, "Pos"=w2599) -> ("delpos"=w2598:dbl[])  [unwired: 1 in, 1 out]
          n561 = Less?(x=w2595, y="Mouse YStop") -> (x < y?=w2593:bool)
          n562 = local write "deltapos"(w2598) -> ()
          n563 = Wait (ms)(milliseconds to wait=u32 10) -> ()  [unwired: 1 out]
        }
      }
      frame #6 {
        n564 = local write "Manual position control"(TRUE ("Manual position control")) -> ()
        n565 = local write "End Wheel"(FALSE ("End Wheel")) -> ()
      }
      frame #7 {
        n566 = while {
          stop <- FALSE stop-if-true
          n567 = Wait (ms)(milliseconds to wait=u32 100) -> ()  [unwired: 1 out]
        }
      }
    }
  }
  n568 = while {
    stop <- FALSE stop-if-true
    n569 = flat-sequence {
      frame #0 {
        n570 = while {
          shift-right: [w2759] -> _
          shift-left: _ -> [w2758]
          stop <- w2757 stop-if-true
          n571 = local read "Number of laps"() -> (w2759:i16)
          n572 = Wait (ms)(milliseconds to wait=u32 250) -> ()  [unwired: 1 out]
          n573 = Greater?(x=w2759, y=w2758) -> (0:w2757:bool)
        }
      }
      frame #1 {
        n574 = local write "Manual \npulse high"(TRUE ("Manual \npulse high")) -> ()
        n575 = Wait (ms)(milliseconds to wait=u32 10) -> ()  [unwired: 1 out]
      }
      frame #2 {
        n576 = Wait (ms)(milliseconds to wait=u32 4000) -> ()  [unwired: 1 out]
      }
      frame #3 {
        n577 = local write "Manual \npulse high"(FALSE ("Manual \npulse high")) -> ()
        n578 = Wait (ms)(milliseconds to wait=u32 10) -> ()  [unwired: 1 out]
      }
    }
    n579 = Wait (ms)(milliseconds to wait=u32 250) -> ()  [unwired: 1 out]
  }
  n580 = while {
    shift-right: ["Close file and open new file"] -> _
    shift-left: _ -> [w2771]
    stop <- FALSE stop-if-true
    n581 = Wait (ms)(milliseconds to wait=u32 100) -> ()  [unwired: 1 out]
    n582 = Greater?(x="Close file and open new file", y=w2771) -> (0:w2769:bool)
    n583 = case shown="True" w2769 {
      tunnel: [FALSE TRUE] -> w2768
      frame False {
      }
      frame True {
        n584 = local write "Close file and open new file"(FALSE ("Close file and open new file")) -> ()
      }
    }
    n585 = Or(x=w2768, y="Stop raspberry pi") -> (x .or. y?=w2766:bool)
    n586 = shared-variable "RT CompactRIO Target\\Mod6\\DIO12"("Record to current file") -> ()  [unwired: 1 in, 1 out]
    n587 = shared-variable "RT CompactRIO Target\\Mod6\\DIO10"("Stop raspberry pi") -> ()  [unwired: 1 in, 1 out]
    n588 = shared-variable "RT CompactRIO Target\\Mod6\\DIO11"(w2766) -> ()  [unwired: 1 in, 1 out]
  }
  n589 = while {
    stop <- FALSE stop-if-true
    n590 = Wait (ms)(milliseconds to wait=u32 250) -> ()  [unwired: 1 out]
    n591 = shared-variable "RT CompactRIO Target\\Mod1\\DI2"() -> (w2779:bool)  [unwired: 1 in, 1 out]
    n592 = shared-variable "RT CompactRIO Target\\Mod1\\DI3"() -> (w2778:bool)  [unwired: 1 in, 1 out]
    n593 = shared-variable "RT CompactRIO Target\\Mod1\\DI0"() -> (w2781:bool)  [unwired: 1 in, 1 out]
    n594 = shared-variable "RT CompactRIO Target\\Mod1\\DI1"() -> (w2780:bool)  [unwired: 1 in, 1 out]
    n595 = Not(x=w2779) -> (.not. x?=w2783:bool)
    n596 = Not(x=w2778) -> (.not. x?=w2782:bool)
    n597 = Not(x=w2781) -> (.not. x?=w2785:bool)
    n598 = Not(x=w2780) -> (.not. x?=w2784:bool)
    n599 = shared-variable "RT CompactRIO Target\\Mod6\\DIO2"(w2783) -> ()  [unwired: 1 in, 1 out]
    n600 = shared-variable "RT CompactRIO Target\\Mod6\\DIO3"(w2782) -> ()  [unwired: 1 in, 1 out]
    n601 = shared-variable "RT CompactRIO Target\\Mod1\\DO2"(w2779) -> ()  [unwired: 1 in, 1 out]
    n602 = shared-variable "RT CompactRIO Target\\Mod1\\DO3"(w2778) -> ()  [unwired: 1 in, 1 out]
    n603 = shared-variable "RT CompactRIO Target\\Mod6\\DIO0"(w2785) -> ()  [unwired: 1 in, 1 out]
    n604 = shared-variable "RT CompactRIO Target\\Mod6\\DIO1"(w2784) -> ()  [unwired: 1 in, 1 out]
    n605 = shared-variable "RT CompactRIO Target\\Mod1\\DO0"(w2781) -> ()  [unwired: 1 in, 1 out]
    n606 = shared-variable "RT CompactRIO Target\\Mod1\\DO1"(w2780) -> ()  [unwired: 1 in, 1 out]
  }
  n607 = while {
    stop <- FALSE stop-if-true
    n608 = flat-sequence {
      frame #0 {
        n609 = while {
          stop <- "Sound" stop-if-true
          n610 = Wait (ms)(milliseconds to wait=u32 250) -> ()  [unwired: 1 out]
        }
      }
      frame #1 {
        n611 = shared-variable "RT CompactRIO Target\\Mod6\\DIO17"(FALSE ("DIO17")) -> ()  [unwired: 1 in, 1 out]
        n612 = Wait (ms)(milliseconds to wait=u32 2000) -> ()  [unwired: 1 out]
      }
      frame #2 {
        n613 = Wait (ms)(milliseconds to wait=u32 100) -> ()  [unwired: 1 out]
        n614 = shared-variable "RT CompactRIO Target\\Mod6\\DIO17"(TRUE ("DIO17")) -> ()  [unwired: 1 in, 1 out]
        n615 = local write "Sound"(FALSE ("Sound")) -> ()
      }
    }
    n616 = Wait (ms)(milliseconds to wait=u32 10) -> ()  [unwired: 1 out]
  }
